vi "MegaAwesome_9_26_12a_JW.vi"() -> ()   [LabVIEW 2011]
uses:
  data/MegaAwesome_States.ctl
  <vilib>/Utility/inputDevices.llb/keyboardAcquire.vi
  <vilib>/Utility/file.llb/Read From Spreadsheet File (string).vi
  <vilib>/Utility/file.llb/Write To Spreadsheet File (string).vi
panel:
  out "Image Center X":i32
  in  "Disable Flag":bool
  out "Index":string
  out "ROI Descriptor out":T1 {"Contours"."Type" items=["No Selection", "Point", "Line", "Rectangle", "Oval", "Polygon", "Freehand Region", "Annulus", "Unused2", "Unused3", "Broken Line", "Freehand Line", "Rotated Rectangle"]}
  out "ROI Descriptor":T1 {"Contours"."Type" items=["No Selection", "Point", "Line", "Rectangle", "Oval", "Polygon", "Freehand Region", "Annulus", "Unused2", "Unused3", "Broken Line", "Freehand Line", "Rotated Rectangle"]}
  in  "Slider Min":dbl=5.0
  in  "Slider Max":dbl=5.0
  out "Opj X Axis":string
  out "X Axis Display Type":string
  in  "Index-Sat":dbl=5.0
  in  "Index-Lin":dbl=5.0
  in  "IndexLog-Lin":dbl=5.0
  in  "IndexLog-Sat":dbl=5.0 caption="Num Pts"
  out "Lin Id-Log Used":dbl[](array[numeric])
  out "Lin-Vg Array-Log Used":dbl[](array[numeric])
  in  "New: Comments":string
  out "Save Array":string[][](array[string])
  out "Folder Index":i32 caption="Length"
  out "Sat Id-Used":dbl[](array[numeric])
  out "Sat Vg Array-Used":dbl[](array[numeric])
  out "Vg Array-Log-Used":dbl[](array[numeric])
  out "Sat Id-Log-Used":dbl[](array[numeric])
  out "Lin Id-Used":dbl[](array[numeric])
  out "Lin-Vg Array-Used":dbl[](array[numeric])
  out "Lin Vd":dbl
  out "Recorded Prop":T2
  out "Current State":T3
  in  "Main Tab Control":T4(tab)
  in  "OE Link":bool
  in  "Transfer File":path
  out "Transfer Folder":path
  in  "1) Transport":bool caption="2) Transport"
  in  "Image Analysis":bool caption="1) Image Analysis"
  in  "Transport\nFolder":path caption="Transport Folder"
  out "Transport\nFile":path=path "D:/UserData/Desktop/Jeremy/WFU/Research/Programs/VI mods/Image Not Found.png" caption="Transport File"
  in  "Image Folder":path
  out "Image File":path=path "D:/UserData/Desktop/Jeremy/WFU/Research/Programs/VI mods/Image Not Found.png"
  out "Fabrication Prop":T5
  out "Distances":dbl[](array[numeric])
  in  "Zoom":i16(slide)=-3 scale=-5.0..5.0
  in  "Magnification":u16(ring) items=["5x", "10x", "20x", "50x", "80x"]
  in  "Undo Button":bool
  in  "Remove Button":bool
  in  "Transfer Plots":T6(tab)=enum."Saturation"
  in  "Lin-Trans Slider":dbl(slide) step=1.0 scale=-2.0..2.0 scale format="%#_1p"
  out "Sqrt-Lin":cluster{dbl[], dbl[]}[](graph)
  in  "Sat-Trans Slider":dbl(slide) step=1.0 scale=-2.0..2.0 scale format="%#_1p"
  out "Sqrt-Sat":cluster{dbl[], dbl[]}[](graph)
  out "Raw- Lin":cluster{dbl[], dbl[]}[](graph)
  out "Raw- Sat":cluster{dbl[], dbl[]}[](graph)
  in  "Log Plots":enum32{"Linear", "Saturation", "Transport"}(tab)=enum."Saturation"
  in  "Lin-Log Slider":dbl(slide) step=1.0 scale=-2.0..2.0 scale format="%#_1p"
  out "Lin-Log":cluster{dbl[], dbl[]}[](graph)
  in  "Sat-Log Slider":dbl(slide) step=1.0 scale=-2.0..2.0 scale format="%#_1p"
  out "Sat-Log":cluster{dbl[], dbl[]}[](graph)
  out "Transport":cluster{dbl[], dbl[]}[](graph)
  out "Transport Name:":string
  in  "Manual Controls":T7
  in  "File Controls":T8
  out "Date Recorded":string="Date Recorded" caption="Measured"
  out "Data Name:":string
  out "Image Name":string
  out "Date Created":string caption="Fabricated"
  in  "Comments:":string
  out "Rec: Length":dbl caption="Length" format="%#_3g"
  out "Rec: Width":dbl caption="Width" format="%#_4g"
  out "Rec: Dielectric (d)":dbl caption="Dielectric (d)" format="%#_3g"
  in  "New: Dielectric":dbl
  in  "New: Length":dbl
  in  "New: Width":dbl
  out "Rec: Temp":dbl caption="Sample Temp" format="%.1f"
  in  "New: Temp":dbl format="%.1f"
  out "Image Out":T9(plugin-control)
  in  "Num Pts":dbl=5.0
  in  "Num Pts Log":dbl=5.0 caption="Num Pts"
  out "Recorded Values Cluster":T10
  out "Calculated Values Cluster":T10 caption="Recorded Values Cluster"
  out "Re-Calculated Values Cluster":T10 caption="Recorded Values Cluster"
  in  "Independant Variable:":string(combo)="Length (um):"
  out "Image Preview":T9(plugin-control)
  out "Total Width":dbl
  in  "Index Array":u16(ring) caption="Index" items=["1A", "1A", "1A", "1A", "1A", "1A", "1A", "1A", "1A", "1A", "1A", "1A", "1A", "1A", "1A", "1A", "1A", "1A", "1A", "1A", "1A", "1A", "1A", "1A", "1A", "1A", "1A", "1A", "1A", "1A", "1A", "1A", "1A", "1A", "1A", "1A", "1A"]
  in  "Room Temp":dbl=294.0 caption="Room Temp (K)"
  out "No Image\n File":path=path "\\\\acad1\\physics/Jurchescu-group/JW-PD/Mega Awesome/Image Not Found.png" caption="No Image File"
  out "Origin Project File":path=path "\\\\acad1\\physics/Jurchescu-group/JW-PD/Group Library/Origin Project Files/DeviceData_8_10_12a_JW.opj"
  out "No Transport\n File":path=path "\\\\acad1\\physics/Jurchescu-group/JW-PD/Mega Awesome/No Transport File.txt" caption="No Transport File"
  in  "Transport Style Controls":T11={"Transport Line Size"=1, "Transport Line Color"=16772608} {"Transport Line Size" items=["Extra Small", "Small", "Medium", "Large", "Extra Large"]}
  out "Application Directory":path
  # "1)  Select the Transfer File that you would like to analyze:"
  # "Transfer Location"
  # "2) What else would you like to view during your analysis?"
  # "Transport Location"
  # "Image Location"
  # "Recorded"
  # "Calculated"
  # "Re-Calculated"
  # "Manual"
  # "um"
  # "Slider\nDoesn't\nWork"
  # "V"
  # "V"
  # "Slider\nDoesn't\nWork"
  # "V"
  # "Default File Choices"
  # "Default Analysis Values"
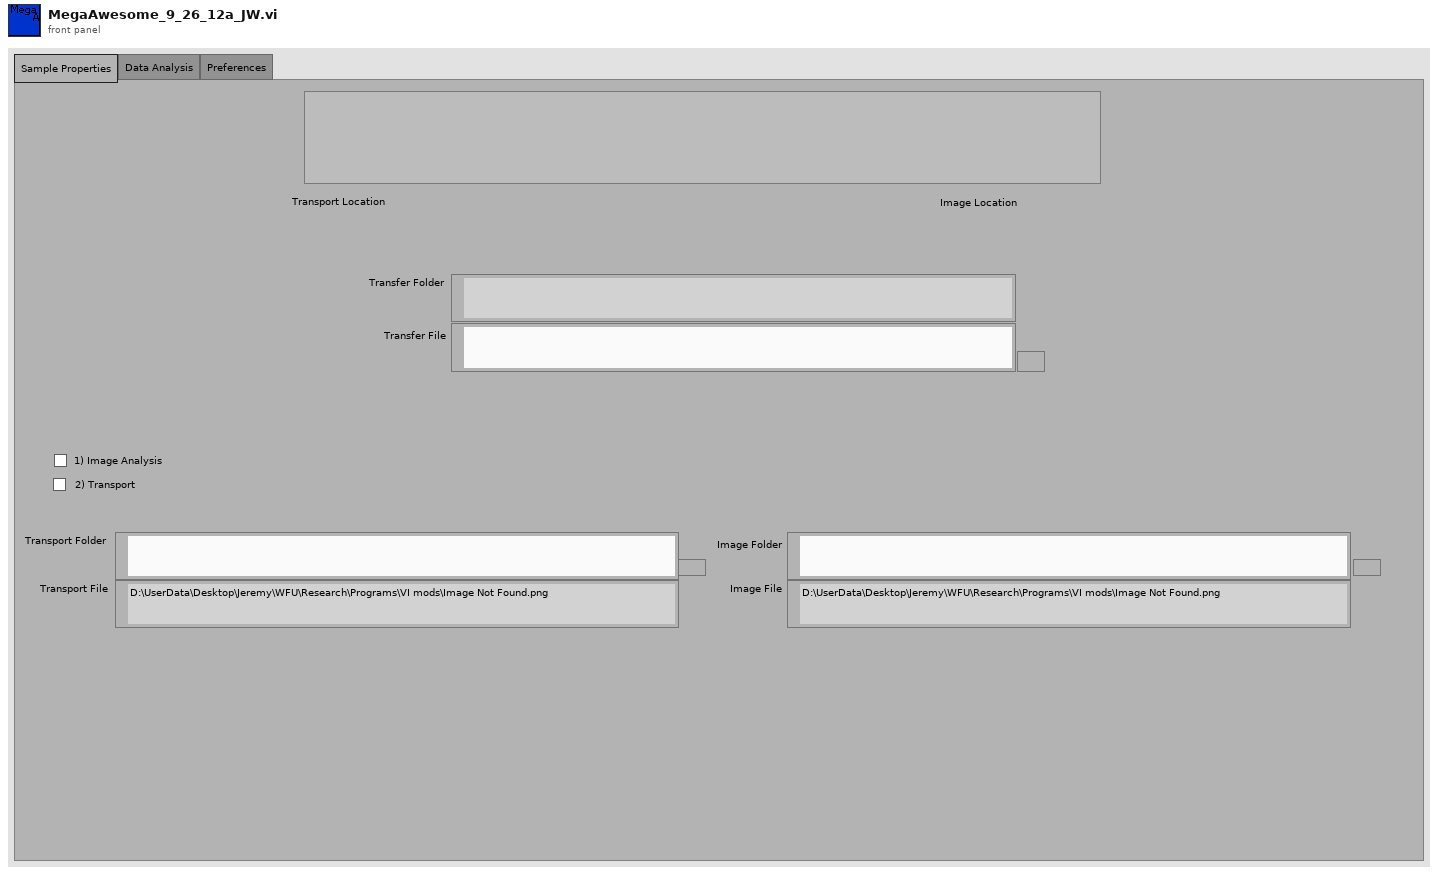
[diagram p1: front panel]
types:
  T1 = typedef "ROI Descriptor" = cluster{"Global Rectangle":i32[], "Contours":cluster{"ID":enum32{"External", "Internal"}, "Type":u32, "Coordinates":i32[]}[]}
  T2 = cluster{"Date Recorded":string, "Index":string, "Length":dbl, "Width":dbl, "Sample Temp":dbl}
  T3 = typedef "MegaAwesome_States.ctl" = enum16{"Init", "File Missing", "No Event", "Read Data", "Calculated Values", "Re-Calculated Values", "Next File", "Previous File", "Discard File", "Save", "Save Lines", "Export", "Exit"}
  T4 = enum32{"Sample Properties", "Data Analysis", "Preferences"}
  T5 = cluster{"Date Created":string, "Material":string, "Solvent":string, "Concentration":dbl, "Method":string, "Dielectric (nm)":dbl, "Treatment":string, "Comments":string}
  T6 = enum32{"Linear", "Saturation", "Raw-Linear", "Raw-Saturation"}
  T7 = cluster{"Manual-Temp":bool, "Manual-Width":bool, "Manuel-Length":bool, "Manuel-Dielectric":bool, "Manual Comments":bool}
  T8 = cluster{"Previous File":bool, "Discard ":bool, "Save Lines":bool, "Close":bool, "Next File ":bool, "Save":bool, "Save Next":bool, "Export":bool}
  T9 = typedef "IMAQ Image.ctl" = refnum<image>
  T10 = cluster{"Mobility-Sat":dbl, "Moblitity-Lin":dbl, "On/Off":dbl, "Off Current":dbl, "Vt-Sat":dbl, "STS":dbl, "Trap Density-VT":dbl, "Trap Density-STS":dbl}
  T11 = cluster{"Transport Line Size":u16, "Transport Line Color":u32}
  T12 = typedef "LVBoundsTypeDef.ctl" = cluster{"Width":u32, "Height":u32}
  T13 = cluster{"Global Rectangle":i32[], "Contours":cluster{"Contour Type":u32, "ROI Type":u32, "Points":i32[]}[]}
  T14 = cluster{"Contour Type":u32, "ROI Type":u32, "Points":i32[]}[]
  T15 = cluster{i32[], cluster{"Contour Type":u32, "ROI Type":u32, "Points":i32[]}[]}
  T16 = enum16{"0", "1", "2", "3", "4", "5", "6", "7", "8", "9", "A", "B", "C", "D", "E", "F", "G", "H", "I", "J", "K", "L", "M", "N", "O", "P", "Q", "R", "S", "T", "U", "V", "W", "X", "Y", "Z", "F1", "F2", "F3", "F4", "F5", "F6", "F7", "F8", "F9", "F10", "F11", "F12", "F13", "F14", "F15", "ADD", "BACK", "BACKSLASH", "CAPITAL", "COMMA", "DECIMAL", "DELETE", "DIVIDE", "DOWN", "END", "EQUALS", "ESCAPE", "GRAVE (`)", "HOME", "INSERT", "LBRACKET", "LCONTROL", "LEFT", "L ALT", "LSHIFT", "LWIN", "MINUS", "MULTIPLY", "NEXT", "NUMLOCK", "NUMPAD_0", "NUMPAD_1", "NUMPAD_2", "NUMPAD_3", "NUMPAD_4", "NUMPAD_5", "NUMPAD_6", "NUMPAD_7", "NUMPAD_8", "NUMPAD_9", "PAUSE", "PERIOD", "PRIOR (PG UP)", "RBRACKET", "RCONTROL", "RETURN", "RIGHT", "R ALT", "RSHIFT", "RWIN", "SCROLL", "SEMICOLON", "SLASH", "SPACE", "SUBTRACT", "TAB", "UP", "ENTER (num pad)", "' (quote)"}[]
  T17 = enum16{"0", "1", "2", "3", "4", "5", "6", "7", "8", "9", "A", "B", "C", "D", "E", "F", "G", "H", "I", "J", "K", "L", "M", "N", "O", "P", "Q", "R", "S", "T", "U", "V", "W", "X", "Y", "Z", "F1", "F2", "F3", "F4", "F5", "F6", "F7", "F8", "F9", "F10", "F11", "F12", "F13", "F14", "F15", "ADD", "BACK", "BACKSLASH", "CAPITAL", "COMMA", "DECIMAL", "DELETE", "DIVIDE", "DOWN", "END", "EQUALS", "ESCAPE", "GRAVE (`)", "HOME", "INSERT", "LBRACKET", "LCONTROL", "LEFT", "L ALT", "LSHIFT", "LWIN", "MINUS", "MULTIPLY", "NEXT", "NUMLOCK", "NUMPAD_0", "NUMPAD_1", "NUMPAD_2", "NUMPAD_3", "NUMPAD_4", "NUMPAD_5", "NUMPAD_6", "NUMPAD_7", "NUMPAD_8", "NUMPAD_9", "PAUSE", "PERIOD", "PRIOR (PG UP)", "RBRACKET", "RCONTROL", "RETURN", "RIGHT", "R ALT", "RSHIFT", "RWIN", "SCROLL", "SEMICOLON", "SLASH", "SPACE", "SUBTRACT", "TAB", "UP", "ENTER (num pad)", "' (quote)"}
  T18 = cluster{string, sgl, bool, bool, bool, bool, bool, bool, i32}
  T19 = cluster{i32, cluster{string, sgl, bool, bool, bool, bool, bool, bool, i32}, i32, i32}
  T20 = cluster{"Contour Type":u32, "ROI Type":u32, "Points":i32[]}
  T21 = cluster{"Points[0]":i32, "Points[1]":i32, "Points[2]":i32, "Points[3]":i32, "Points[4]":i32, "Points[5]":i32, "Points[6]":i32, "Points[7]":i32, "Points[8]":i32}
  T22 = cluster{"[0]":cluster{dbl[], dbl[]}, "[1]":cluster{dbl[], dbl[]}, "[2]":cluster{dbl[], dbl[]}, "[3]":cluster{dbl[], dbl[]}, "[4]":cluster{dbl[], dbl[]}, "[5]":cluster{dbl[], dbl[]}, "[6]":cluster{dbl[], dbl[]}, "[7]":cluster{dbl[], dbl[]}, "[8]":cluster{dbl[], dbl[]}}
  T23 = cluster{"Sat Vg Used":dbl[], "Sat Sqrt(Id) Used ":dbl[], "Lin Vg Used":dbl[], "Lin Sqrt(Id) Used":dbl[], "Index-Lin":dbl, "Index-Sat":dbl}
  T24 = cluster{"Raw Sat":cluster{dbl[], dbl[]}[], "Sqrt Sat":cluster{dbl[], dbl[]}[], "Log Sat":cluster{dbl[], dbl[]}[], "Raw Lin":cluster{dbl[], dbl[]}[], "Sqrt Lin":cluster{dbl[], dbl[]}[], "Log Lin":cluster{dbl[], dbl[]}[]}
  T25 = cluster{"Mobility-Sat":dbl, "Vt-Sat":dbl, "Mobility-Lin":dbl, "Vt-Lin":dbl, "Off I-Sat":dbl, "On/Off I-Sat":dbl}
  T26 = cluster{"Sat Vg Used":dbl[], "Sat Log(Id) Used":dbl[], "Lin Vg Used":dbl[], "Lin Log(Id) Used":dbl[], "STS Index-Sat":dbl, "STS Index-Lin":dbl}
  T27 = cluster{"Independant  Variable Indicator":string, "Parameter String Indicator":string}
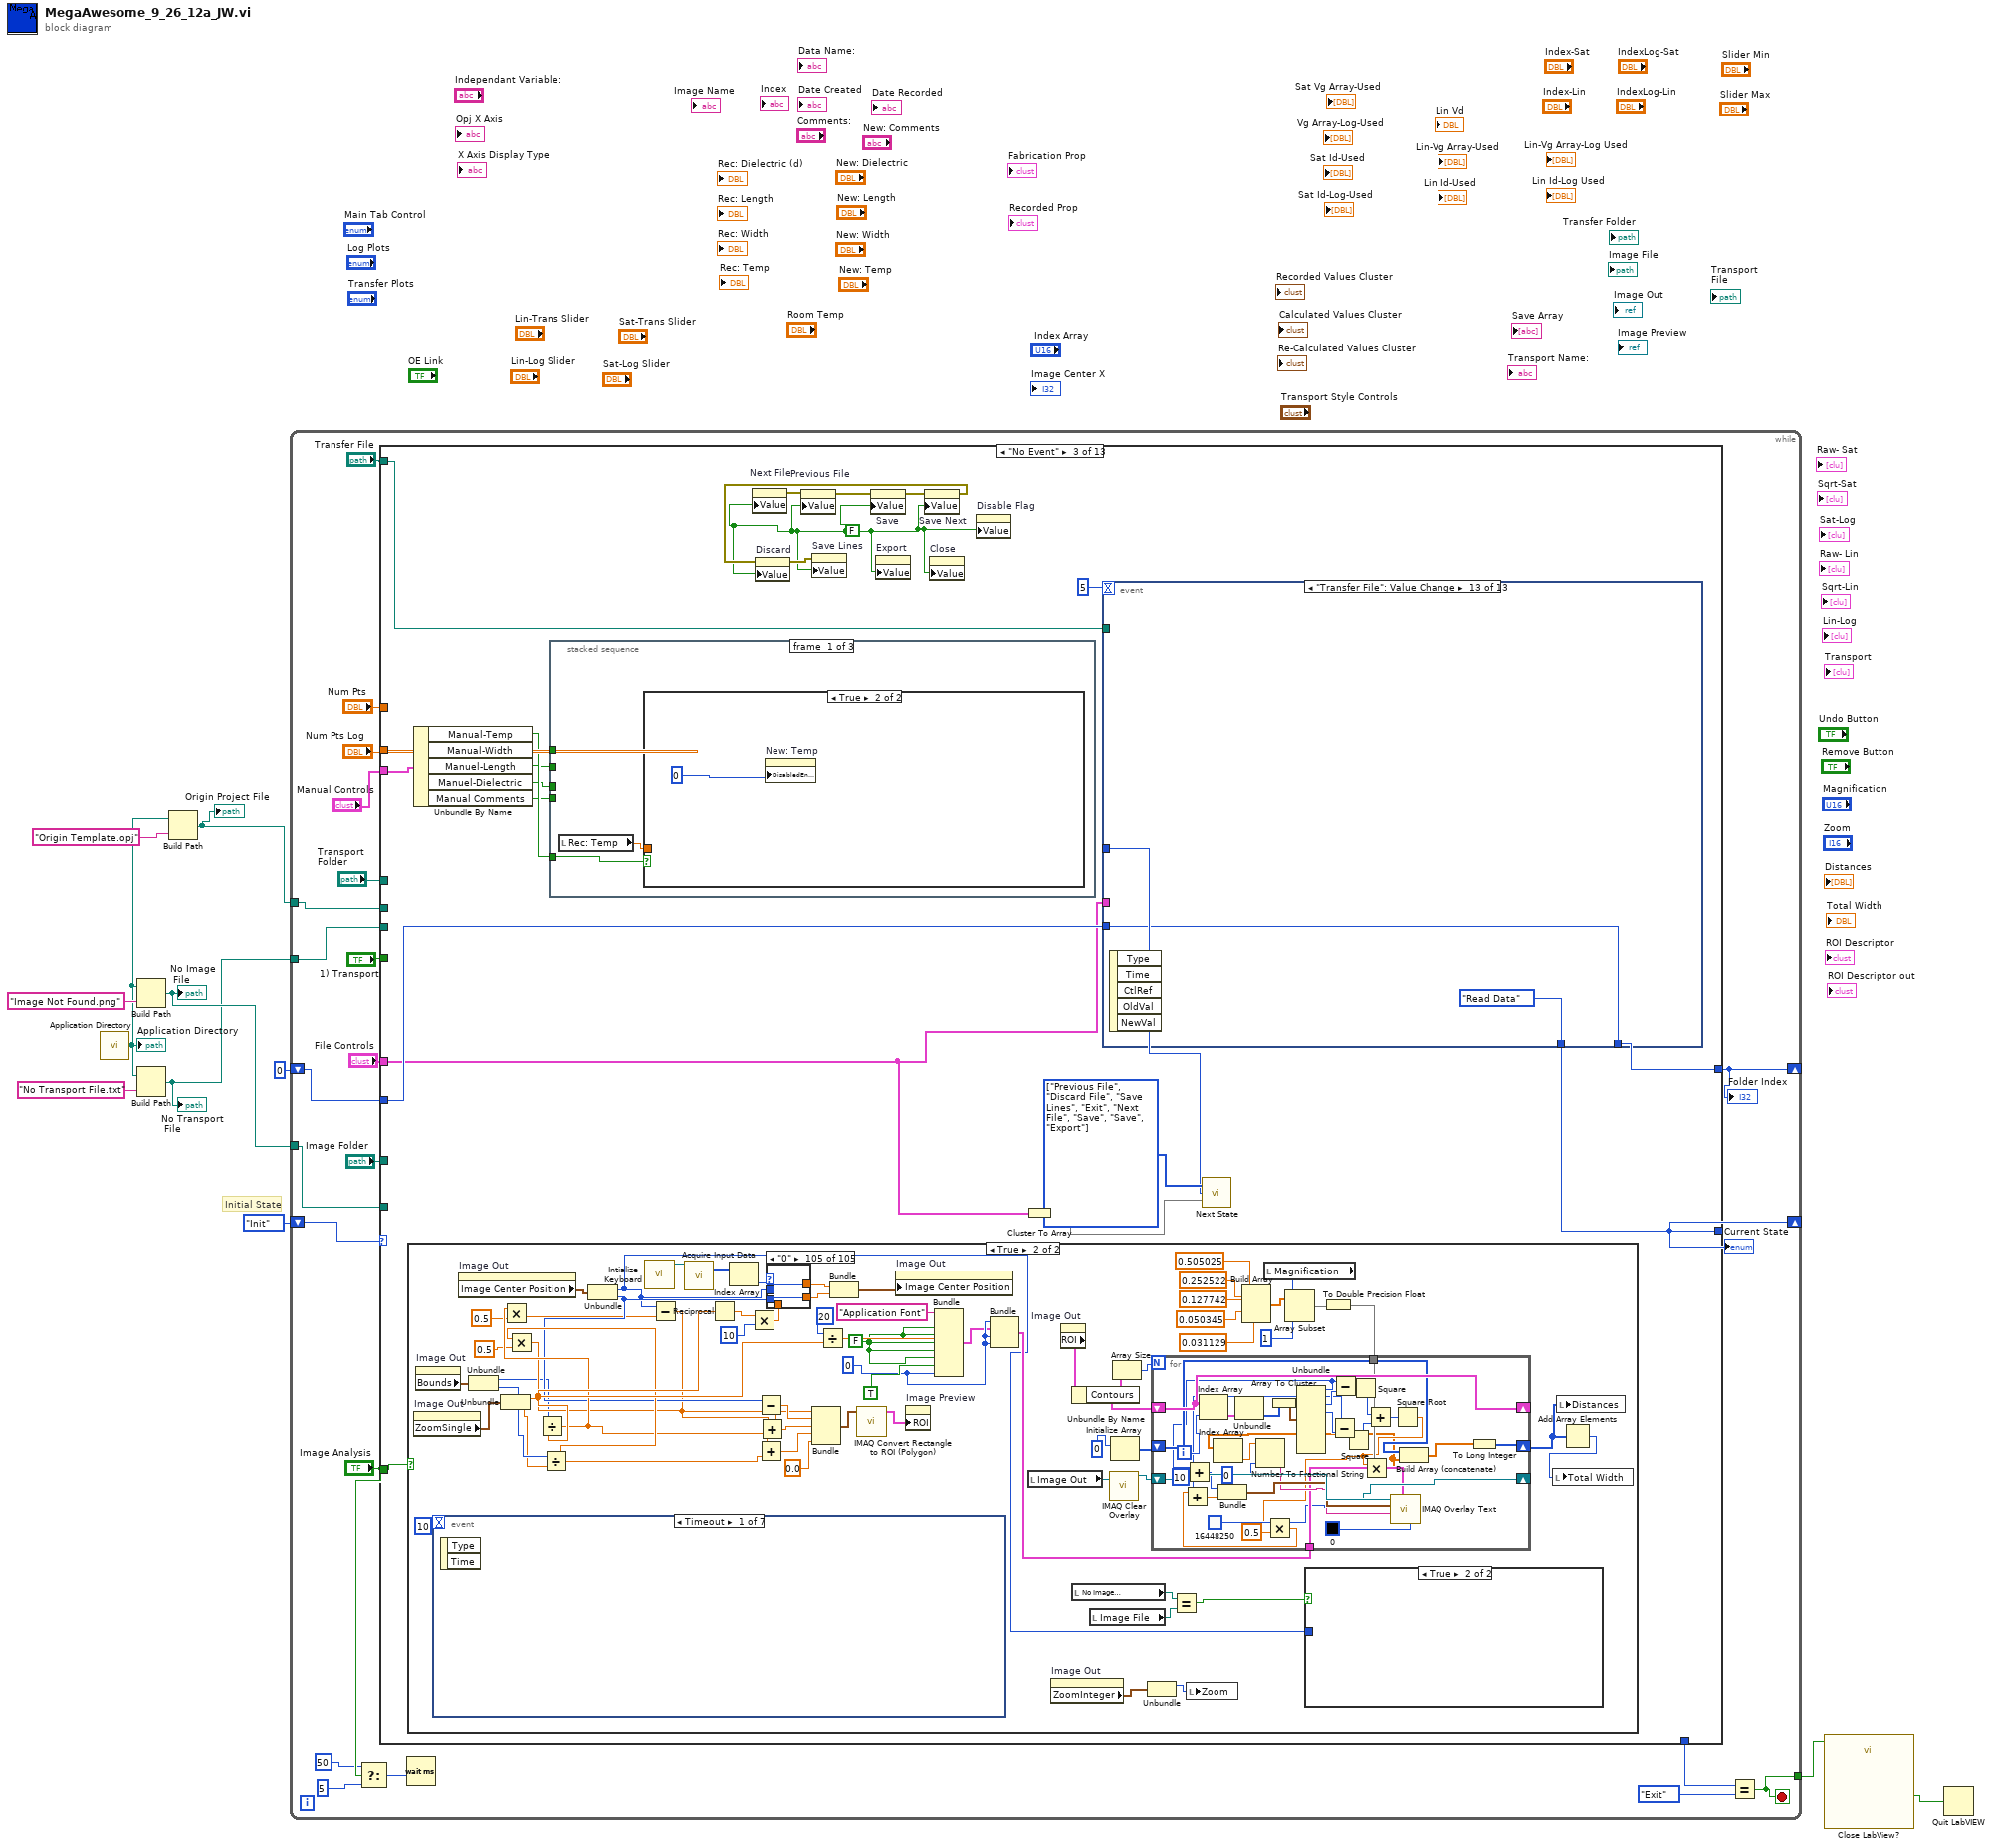
[diagram p0: block diagram]
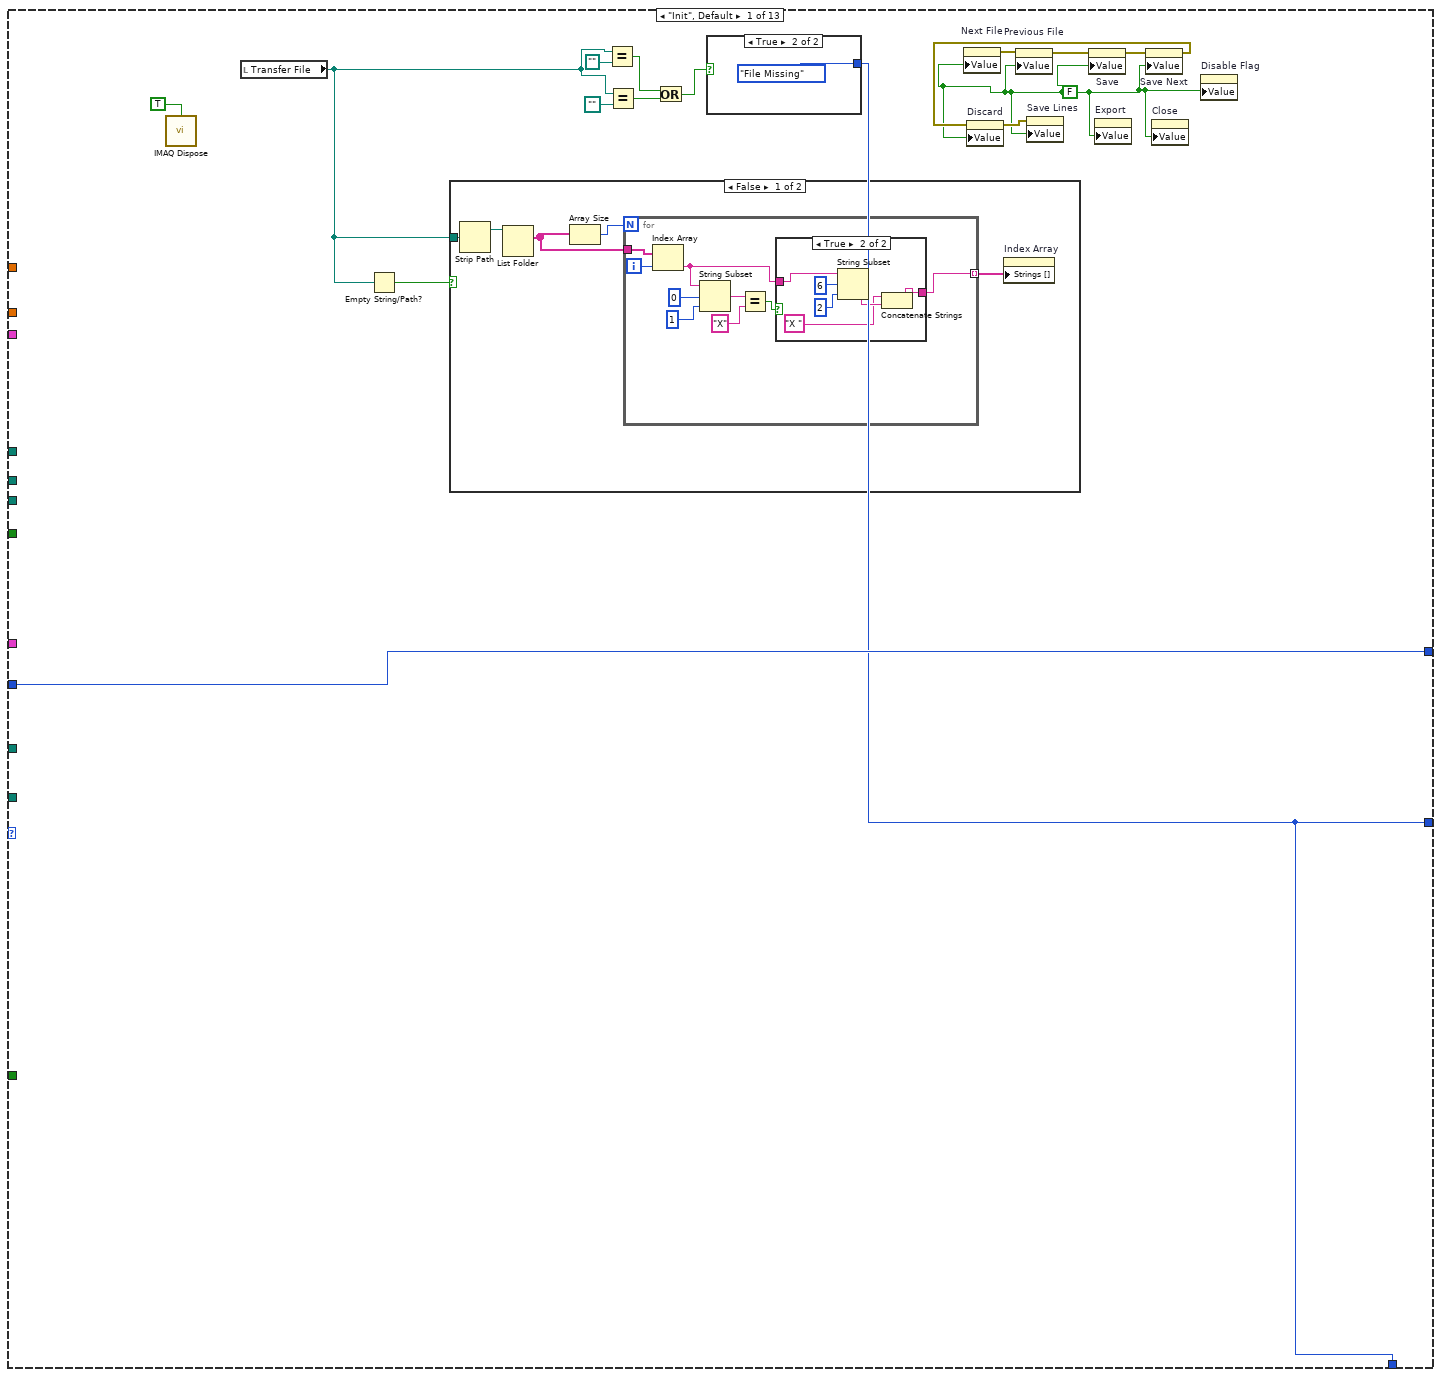
[diagram p2: hidden frame]
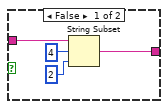
[diagram p3: hidden frame]
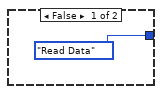
[diagram p5: hidden frame]
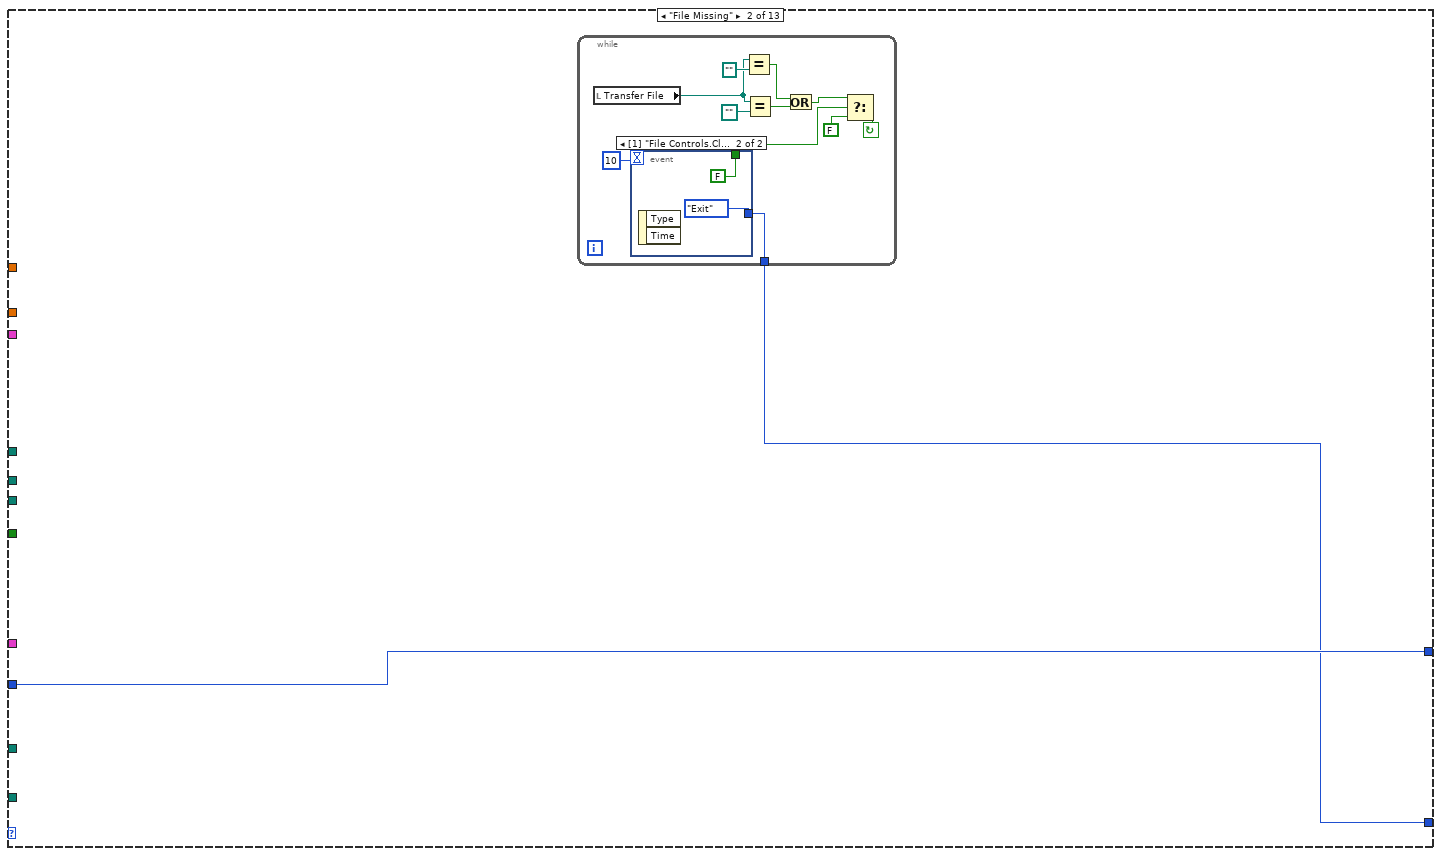
[diagram p6: hidden frame]
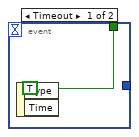
[diagram p7: hidden frame]
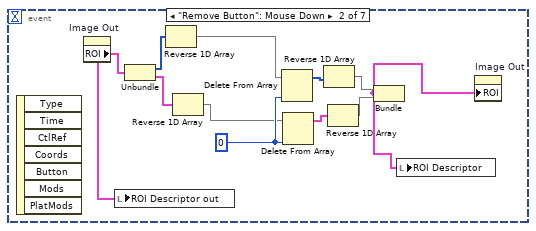
[diagram p9: hidden frame]
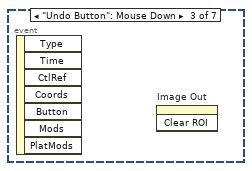
[diagram p10: hidden frame]
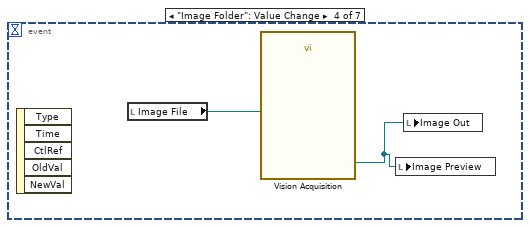
[diagram p11: hidden frame]
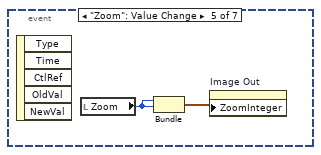
[diagram p12: hidden frame]
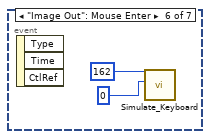
[diagram p13: hidden frame]
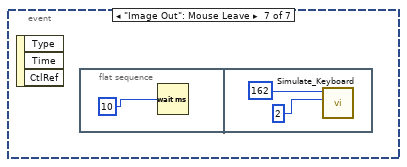
[diagram p14: hidden frame]
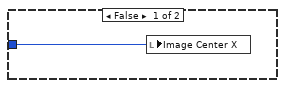
[diagram p15: hidden frame]
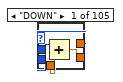
[diagram p16: hidden frame]
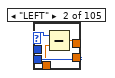
[diagram p17: hidden frame]
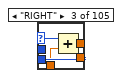
[diagram p18: hidden frame]
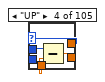
[diagram p19: hidden frame]
diagram:
  # "Initial State"
  n1 = call <vilib>:"Application Directory.vi"() -> ("Application Directory"=w4:path)
  "Application Directory" <- w4
  n2 = Build Path(base path=w4, name or relative path="Image Not Found.png") -> (appended path=w7:path)
  "No Image\n File" <- w7
  n3 = Build Path(base path=w4, name or relative path="No Transport File.txt") -> (appended path=w6:path)
  "No Transport\n File" <- w6
  n4 = Build Path(base path=w4, name or relative path="Origin Template.opj") -> (appended path=w5:path)
  "Origin Project File" <- w5
  n5 = while {
    shift-right: [w15] -> _
    shift-left: MegaAwesome_States."Init" -> [w13]
    shift-right: [w27] -> _
    shift-left: 0 -> [w28]
    tunnel: w7 -> [w19]
    tunnel: w6 -> [w17]
    tunnel: w5 -> [w16]
    tunnel: [w14] -> w2
    stop <- w14 stop-if-true
    n6 = Select(t=50, s="Image Analysis", f=5) -> (s? t:f=w21:i32)
    n7 = case shown="\"No Event\"" w13 {
      tunnel: [w34 w76 w104 MegaAwesome_States."Calculated Values" MegaAwesome_States."Re-Calculated Values" MegaAwesome_States."No Event" MegaAwesome_States."Read Data" MegaAwesome_States."Read Data" MegaAwesome_States."Init" w839 w1360 MegaAwesome_States."No Event" MegaAwesome_States."Exit"] -> w15
      tunnel: "Transfer File" -> [_ _ w94 w612 w659 _ w780 w791 w809 w844 _ _ _]
      tunnel: "Num Pts" -> [_ _ _ _ w683 _ _ _ _ _ _ _ _]
      tunnel: "Num Pts Log" -> [_ _ _ _ w682 _ _ _ _ _ _ _ _]
      tunnel: "Image Folder" -> [_ _ _ _ w679 _ _ _ _ _ _ w1371 _]
      tunnel: w19 -> [_ _ _ _ w678 _ _ _ _ _ _ _ _]
      tunnel: [w44 w77 w95 w617 w677 w740 w766 w789 w804 w845 w1361 w1381 w1386] -> w27
      tunnel: w28 -> [w44 w77 w96 w615 w677 w740 w767 w790 _ w845 w1361 w1381 w1386]
      tunnel: "Manual Controls" -> [_ _ w106 _ _ _ _ _ _ w843 _ _ _]
      tunnel: "File Controls" -> [_ _ w92 _ _ _ _ _ _ w838 _ _ _]
      tunnel: "1) Transport" -> [_ _ _ _ w650 _ _ _ _ _ _ _ _]
      tunnel: "Image Analysis" -> [_ _ w97 _ w649 _ _ _ _ _ _ _ _]
      tunnel: "Transport\nFolder" -> [_ _ _ _ w648 _ _ _ _ _ _ _ _]
      tunnel: w17 -> [_ _ _ _ w647 _ _ _ _ _ _ _ _]
      tunnel: w16 -> [_ _ _ _ _ _ _ _ _ _ _ _ w1385]
      tunnel: [w34 _ _ _ _ _ _ _ _ _ w1359 _ _] -> w12
      frame "Init", Default {
        w35 = FALSE
        n8 = call "IMAQ Dispose"("All Images? (No)"=TRUE) -> ()  [unwired: 5 in, 1 out]
        n9 = local read "Transfer File"() -> (w42:path)
        n10 = Empty String/Path?(string/path=w42) -> (empty?=w43:bool)
        n11 = case shown="False" w43 {
          tunnel: w42 -> [w51 _]
          frame False {
            n12 = Strip Path(path=w51) -> (stripped path=w53:path)  [unwired: 1 out]
            n13 = List Folder(path=w53) -> (filenames=w52:string[])  [unwired: 3 in, 3 out]
            n14 = Array Size(array=w52) -> (size(s)=w54:i32)
            n15 = for {
              N: w54 -> [_]
              tunnel: w52 -> [w63]
              tunnel: [w61] -> w50 mode=indexing
              i -> [w62]
              n16 = Index Array(array=w63, index=w62) -> (element=w60:string)
              n17 = String Subset(string=w60, offset (0)=0, length (rest)=1) -> (substring=w57:string)
              n18 = Equal?(x=w57, y="X") -> (x = y?=w56:bool)
              n19 = case shown="True" w56 {
                tunnel: w60 -> [w67 w71]
                tunnel: [w64 w70] -> w61
                frame False {
                  n20 = String Subset(string=w67, offset (0)=4, length (rest)=2) -> (substring=w64:string)
                }
                frame True {
                  n21 = String Subset(string=w71, offset (0)=6, length (rest)=2) -> (substring=w69:string)
                  n22 = Concatenate Strings("X ", w69) -> (w70:string)
                }
              }
            }
            n23 = property on="Index Array" class="Ring (strict)"("Strings []"=w50) -> ()  [unwired: 2 in, 2 out]
          }
          frame True {
          }
        }
        n24 = Equal?(x=w42, y=path "") -> (x = y?=w47:bool)
        n25 = Equal?(x=w42, y=path "") -> (x = y?=w46:bool)
        n26 = Or(x=w47, y=w46) -> (x .or. y?=w49:bool)
        n27 = case shown="True" w49 {
          tunnel: [MegaAwesome_States."Read Data" MegaAwesome_States."File Missing"] -> w34
          frame False {
          }
          frame True {
          }
        }
        n28 = property on="Next File" class="Bool (strict)"("Value"=w35) -> (error out=w40:errorcluster)  [unwired: 2 in, 1 out]
        n29 = property on="Previous File" class="Bool (strict)"(error in=w40, "Value"=w35) -> (error out=w39:errorcluster)  [unwired: 1 in, 1 out]
        n30 = property on="Save" class="Bool (strict)"(error in=w39, "Value"=w35) -> (error out=w38:errorcluster)  [unwired: 1 in, 1 out]
        n31 = property on="Export" class="Bool (strict)"("Value"=w35) -> ()  [unwired: 2 in, 2 out]
        n32 = property on="Save Next" class="Bool (strict)"(error in=w38, "Value"=w35) -> (error out=w37:errorcluster)  [unwired: 1 in, 1 out]
        n33 = property on="Discard" class="Bool (strict)"(error in=w37, "Value"=w35) -> (error out=w36:errorcluster)  [unwired: 1 in, 1 out]
        n34 = property on="Save Lines" class="Bool (strict)"(error in=w36, "Value"=w35) -> ()  [unwired: 1 in, 2 out]
        n35 = property on="Close" class="Bool (strict)"("Value"=w35) -> ()  [unwired: 2 in, 2 out]
        n36 = property on="Disable Flag" class="Bool (strict)"("Value"=w35) -> ()  [unwired: 2 in, 2 out]
      }
      frame "File Missing" {
        n37 = while {
          tunnel: [w83] -> w76
          stop <- w79 continue-if-true
          n38 = local read "Transfer File"() -> (w84:path)
          n39 = event shown="[1] \"File Controls.Close\": Value Change" {
            selector: _ -> [_ _]
            dyn-events: _ -> [_ _]
            timeout: 10 -> [_ _]
            tunnel: [_ MegaAwesome_States."Exit"] -> w83
            tunnel: [TRUE FALSE] -> w82
            event Timeout {
              n40 = event-data() -> ()  [unwired: 1 in, 2 out]
            }
            event "File Controls.Close": Value Change {
              n41 = event-data() -> ()  [unwired: 1 in, 2 out]
            }
          }
          n42 = Equal?(x=w84, y=path "") -> (x = y?=w86:bool)
          n43 = Equal?(x=w84, y=path "") -> (x = y?=w87:bool)
          n44 = Or(x=w86, y=w87) -> (x .or. y?=w81:bool)
          n45 = Select(t=w81, s=w82, f=FALSE) -> (s? t:f=w79:bool)
        }
      }
      frame "No Event" {
        w93 = FALSE
        w113 = T3[] [enum."Previous File", enum."Discard File", enum."Save Lines", enum."Exit", enum."Next File", enum."Save", enum."Save", enum."Export"] items=["Init", "File Missing", "No Event", "Read Data", "Calculated Values", "Re-Calculated Values", "Next File", "Previous File", "Discard File", "Save", "Save Lines", "Export", "Exit"]
        n46 = case shown="True" w97 {
          frame False {
          }
          frame True {
            w169 = FALSE
            w171 = 0
            n47 = property on="Image Out" class="ImageControl"() -> ("ZoomSingle"=w155:cluster{"X":sgl, "Y":sgl})  [unwired: 2 in, 2 out]
            n48 = property on="Image Out" class="ImageControl"() -> ("Bounds"=w154:T12)  [unwired: 2 in, 2 out]
            n49 = event shown="[0] Timeout" {
              selector: _ -> [_ _ _ _ _ _ _]
              dyn-events: _ -> [_ _ _ _ _ _ _]
              timeout: 10 -> [_ _ _ _ _ _ _]
              event Timeout {
                n50 = event-data() -> ()  [unwired: 1 in, 2 out]
              }
              event "Remove Button": Mouse Down {
                w188 = 0
                n51 = event-data() -> ()  [unwired: 1 in, 7 out]
                n52 = property on="Image Out" class="ImageControl"() -> ("ROI"=w178:T13)  [unwired: 2 in, 2 out]
                n53 = local write "ROI Descriptor out"(w178) -> ()
                n54 = Unbundle(w178) -> ("Global Rectangle"=w187:i32[], "Contours"=w185:T14)
                n55 = Reverse 1D Array(array=w187) -> (reversed array=w186:i32[])
                n56 = Reverse 1D Array(array=w185) -> (reversed array=w184:T14)
                n57 = Delete From Array(array=w186, index=w188) -> (array with subset deleted=w183:i32[])  [unwired: 1 in, 1 out]
                n58 = Delete From Array(array=w184, index=w188) -> (array with subset deleted=w182:T14)  [unwired: 1 in, 1 out]
                n59 = Reverse 1D Array(array=w183) -> (reversed array=w181:i32[])
                n60 = Reverse 1D Array(array=w182) -> (reversed array=w180:T14)
                n61 = Bundle(w181, w180) -> (w179:T15)  [unwired: 1 in]
                n62 = local write "ROI Descriptor"(w179) -> ()
                n63 = property on="Image Out" class="ImageControl"("ROI"=w179) -> ()  [unwired: 2 in, 2 out]
              }
              event "Undo Button": Mouse Down {
                n64 = event-data() -> ()  [unwired: 1 in, 7 out]
                n65 = invoke on="Image Out" class="ImageControl" method="Clear ROI"() -> ()  [unwired: 3 in, 3 out]
              }
              event "Image Folder": Value Change {
                n66 = event-data() -> ()  [unwired: 1 in, 5 out]
                n67 = local read "Image File"() -> (w190:path)
                n68 = call "Vision Acquisition"("Image Path"=w190) -> ("Image Out"=w189:T9)  [unwired: 25 in, 1 out]
                n69 = local write "Image Preview"(w189) -> ()
                n70 = local write "Image Out"(w189) -> ()
              }
              event "Zoom": Value Change {
                n71 = event-data() -> ()  [unwired: 1 in, 5 out]
                n72 = local read "Zoom"() -> (w191:i16)
                n73 = Bundle("Zoom"=w191, "Zoom"=w191) -> (w192:cluster{"Zoom":i16, "Zoom":i16})  [unwired: 1 in]
                n74 = property on="Image Out" class="ImageControl"("ZoomInteger"=w192) -> ()  [unwired: 2 in, 2 out]
              }
              event "Image Out": Mouse Enter {
                n75 = event-data() -> ()  [unwired: 1 in, 3 out]
                n76 = call "Simulate_Keyboard.vi"("Action"=0, "Virtual Key"=162) -> ()  [unwired: 7 in, 1 out]
              }
              event "Image Out": Mouse Leave {
                n77 = event-data() -> ()  [unwired: 1 in, 3 out]
                n78 = flat-sequence {
                  frame #0 {
                    n79 = Wait (ms)(milliseconds to wait=10) -> ()  [unwired: 1 out]
                  }
                  frame #1 {
                    n80 = call "Simulate_Keyboard.vi"("Action"=2, "Virtual Key"=162) -> ()  [unwired: 7 in, 1 out]
                  }
                }
              }
            }
            n81 = property on="Image Out" class="ImageControl"() -> ("Image Center Position"=w148:cluster{"X":u32, "Y":u32})  [unwired: 2 in, 2 out]
            n82 = Unbundle(w154) -> ("Width"=w157:u32, "Height"=w158:u32)
            n83 = Unbundle(w155) -> ("X"=w175:sgl, "Y"=w156:sgl)
            n84 = Divide(x=w157, y=w175) -> (x/y=w166:sgl)
            n85 = Multiply(x=w166, y=0.5) -> (x*y=w161:dbl)
            n86 = Divide(x=w158, y=w156) -> (x/y=w167:sgl)
            n87 = Multiply(x=w167, y=0.5) -> (x*y=w162:dbl)
            n88 = Unbundle(w148) -> ("X"=w118:u32, "Y"=w165:u32)
            n89 = call <vilib>:"Intialize Keyboard.vi"() -> ("device ID"=w145:refnum<k1>)  [unwired: 10 in, 1 out]
            n90 = Subtract(x=w118, y=w161) -> (x-y=w163:dbl)
            n91 = call-poly <vilib>:"Acquire Input Data.vi"("device ID"=w145) -> ("keys pressed"=w146:T16)  [unwired: 16 in, 2 out]
            n92 = Reciprocal(x=w175) -> (1/x=w176:sgl)
            n93 = Index Array(array=w146) -> (element=w142:T17)  [unwired: 1 in]
            n94 = Multiply(x=w176, y=10) -> (x*y=w174:sgl)
            n95 = Subtract(x=w165, y=w162) -> (x-y=w164:dbl)
            n96 = Add(x=w164, y=w167) -> (x+y=w150:dbl)
            n97 = Add(x=w163, y=w166) -> (x+y=w149:dbl)
            n98 = case shown="\"0\"" w142 {
              tunnel: w118 -> [w234 w240 w244 w246 w250 w252 w254 w256 w258 w260 w262 w264 w266 w268 w270 w272 w274 w276 w278 w280 w282 w284 w286 w288 w290 w292 w294 w296 w298 w300 w302 w304 w306 w308 w310 w312 w314 w316 w318 w320 w322 w324 w326 w328 w330 w332 w334 w336 w338 w340 w342 w344 w346 w348 w350 w352 w354 w356 w358 w360 w362 w364 w366 w368 w370 w372 w374 w376 w378 w380 w382 w384 w386 w388 w390 w392 w394 w396 w398 w400 w402 w404 w406 w408 w410 w412 w414 w416 w418 w420 w422 w424 w426 w428 w430 w432 w434 w436 w438 w440 w442 w444 w446 w448 w450]
              tunnel: [w234 w239 w243 w246 w250 w252 w254 w256 w258 w260 w262 w264 w266 w268 w270 w272 w274 w276 w278 w280 w282 w284 w286 w288 w290 w292 w294 w296 w298 w300 w302 w304 w306 w308 w310 w312 w314 w316 w318 w320 w322 w324 w326 w328 w330 w332 w334 w336 w338 w340 w342 w344 w346 w348 w350 w352 w354 w356 w358 w360 w362 w364 w366 w368 w370 w372 w374 w376 w378 w380 w382 w384 w386 w388 w390 w392 w394 w396 w398 w400 w402 w404 w406 w408 w410 w412 w414 w416 w418 w420 w422 w424 w426 w428 w430 w432 w434 w436 w438 w440 w442 w444 w446 w448 w450] -> w143
              tunnel: w165 -> [w236 w238 w242 w248 w249 w251 w253 w255 w257 w259 w261 w263 w265 w267 w269 w271 w273 w275 w277 w279 w281 w283 w285 w287 w289 w291 w293 w295 w297 w299 w301 w303 w305 w307 w309 w311 w313 w315 w317 w319 w321 w323 w325 w327 w329 w331 w333 w335 w337 w339 w341 w343 w345 w347 w349 w351 w353 w355 w357 w359 w361 w363 w365 w367 w369 w371 w373 w375 w377 w379 w381 w383 w385 w387 w389 w391 w393 w395 w397 w399 w401 w403 w405 w407 w409 w411 w413 w415 w417 w419 w421 w423 w425 w427 w429 w431 w433 w435 w437 w439 w441 w443 w445 w447 w449]
              tunnel: [w235 w238 w242 w247 w249 w251 w253 w255 w257 w259 w261 w263 w265 w267 w269 w271 w273 w275 w277 w279 w281 w283 w285 w287 w289 w291 w293 w295 w297 w299 w301 w303 w305 w307 w309 w311 w313 w315 w317 w319 w321 w323 w325 w327 w329 w331 w333 w335 w337 w339 w341 w343 w345 w347 w349 w351 w353 w355 w357 w359 w361 w363 w365 w367 w369 w371 w373 w375 w377 w379 w381 w383 w385 w387 w389 w391 w393 w395 w397 w399 w401 w403 w405 w407 w409 w411 w413 w415 w417 w419 w421 w423 w425 w427 w429 w431 w433 w435 w437 w439 w441 w443 w445 w447 w449] -> w144
              tunnel: w174 -> [w233 w237 w241 w245 _ _ _ _ _ _ _ _ _ _ _ _ _ _ _ _ _ _ _ _ _ _ _ _ _ _ _ _ _ _ _ _ _ _ _ _ _ _ _ _ _ _ _ _ _ _ _ _ _ _ _ _ _ _ _ _ _ _ _ _ _ _ _ _ _ _ _ _ _ _ _ _ _ _ _ _ _ _ _ _ _ _ _ _ _ _ _ _ _ _ _ _ _ _ _ _ _ _ _ _ _]
              frame "DOWN" {
                n99 = Add(x=w236, y=w233) -> (x+y=w235:sgl)
              }
              frame "LEFT" {
                n100 = Subtract(x=w240, y=w237) -> (x-y=w239:sgl)
              }
              frame "RIGHT" {
                n101 = Add(x=w244, y=w241) -> (x+y=w243:sgl)
              }
              frame "UP" {
                n102 = Subtract(x=w248, y=w245) -> (x-y=w247:sgl)
              }
              frame "ENTER (num pad)" {
              }
              frame "' (quote)" {
              }
              frame "END" {
              }
              frame "EQUALS" {
              }
              frame "ESCAPE" {
              }
              frame "GRAVE (`)" {
              }
              frame "HOME" {
              }
              frame "INSERT" {
              }
              frame "LBRACKET" {
              }
              frame "LCONTROL" {
              }
              frame "L ALT" {
              }
              frame "LSHIFT" {
              }
              frame "LWIN" {
              }
              frame "MINUS" {
              }
              frame "MULTIPLY" {
              }
              frame "NEXT" {
              }
              frame "NUMLOCK" {
              }
              frame "NUMPAD_0" {
              }
              frame "NUMPAD_1" {
              }
              frame "NUMPAD_2" {
              }
              frame "NUMPAD_3" {
              }
              frame "NUMPAD_4" {
              }
              frame "NUMPAD_5" {
              }
              frame "NUMPAD_6" {
              }
              frame "NUMPAD_7" {
              }
              frame "NUMPAD_8" {
              }
              frame "NUMPAD_9" {
              }
              frame "PAUSE" {
              }
              frame "PERIOD" {
              }
              frame "PRIOR (PG UP)" {
              }
              frame "RBRACKET" {
              }
              frame "RCONTROL" {
              }
              frame "RETURN" {
              }
              frame "R ALT" {
              }
              frame "RSHIFT" {
              }
              frame "RWIN" {
              }
              frame "SCROLL" {
              }
              frame "SEMICOLON" {
              }
              frame "SLASH" {
              }
              frame "SPACE" {
              }
              frame "SUBTRACT" {
              }
              frame "TAB" {
              }
              frame "DIVIDE" {
              }
              frame "DELETE" {
              }
              frame "DECIMAL" {
              }
              frame "COMMA" {
              }
              frame "CAPITAL" {
              }
              frame "BACKSLASH" {
              }
              frame "BACK" {
              }
              frame "ADD" {
              }
              frame "F15" {
              }
              frame "F14" {
              }
              frame "F13" {
              }
              frame "F12" {
              }
              frame "F11" {
              }
              frame "F10" {
              }
              frame "F9" {
              }
              frame "F8" {
              }
              frame "F7" {
              }
              frame "F6" {
              }
              frame "F5" {
              }
              frame "F4" {
              }
              frame "F3" {
              }
              frame "F2" {
              }
              frame "F1" {
              }
              frame "Z" {
              }
              frame "Y" {
              }
              frame "X" {
              }
              frame "W" {
              }
              frame "V" {
              }
              frame "U" {
              }
              frame "T" {
              }
              frame "S" {
              }
              frame "R" {
              }
              frame "Q" {
              }
              frame "P" {
              }
              frame "O" {
              }
              frame "N" {
              }
              frame "M" {
              }
              frame "L" {
              }
              frame "K" {
              }
              frame "J" {
              }
              frame "I" {
              }
              frame "H" {
              }
              frame "G" {
              }
              frame "F" {
              }
              frame "E" {
              }
              frame "D" {
              }
              frame "C" {
              }
              frame "B" {
              }
              frame "A" {
              }
              frame "9" {
              }
              frame "8" {
              }
              frame "7" {
              }
              frame "6" {
              }
              frame "5" {
              }
              frame "4" {
              }
              frame "3" {
              }
              frame "2" {
              }
              frame "1" {
              }
              frame "0" {
              }
            }
            n103 = Bundle(w163, w164, w149, w150, 0.0) -> (w151:cluster{dbl, dbl, dbl, dbl, dbl})  [unwired: 1 in]
            n104 = Divide(x=20, y=w175) -> (x/y=w173:sgl)
            n105 = Bundle("X"=w143, "Y"=w144) -> (w147:cluster{"X":sgl, "Y":sgl})  [unwired: 1 in]
            n106 = call "IMAQ Convert Rectangle to ROI (Polygon)"("Rectangle"=w151) -> ("ROI Descriptor"=w153:T1)  [unwired: 7 in, 2 out]
            n107 = property on="Image Out" class="ImageControl"("Image Center Position"=w147) -> ()  [unwired: 2 in, 2 out]
            n108 = property on="Image Preview" class="ImageControl"("ROI"=w153) -> ()  [unwired: 2 in, 2 out]
            n109 = Bundle("Application Font", w173, w169, w169, w169, w169, w169, TRUE, w171) -> (w168:T18)  [unwired: 1 in]
            n110 = Bundle(w171, w168, w171, w171) -> (w123:T19)  [unwired: 1 in]
            n111 = local read "Image Out"() -> (w122:T9)
            n112 = property on="Image Out" class="ImageControl"() -> ("ZoomInteger"=w121:cluster{"X":i32, "Y":i32})  [unwired: 2 in, 2 out]
            n113 = property on="Image Out" class="ImageControl"() -> ("ROI"=w126:T13)  [unwired: 2 in, 2 out]
            n114 = Unbundle By Name(w126) -> ("Contours"=w127:T14)
            n115 = local read "No Image\n File"() -> (w117:path)
            n116 = local read "Image File"() -> (w116:path)
            n117 = call "IMAQ Clear Overlay"("Image"=w122) -> ("Image Out"=w141:T9)  [unwired: 9 in, 1 out]
            n118 = Initialize Array(0) -> (w129:i32[])  [unwired: 1 in]
            n119 = Array Size(array=w127) -> (size(s)=w128:i32)
            n120 = Unbundle(w121) -> ("X"=w120:i32)  [unwired: 1 out]
            n121 = Equal?(x=w117, y=w116) -> (x = y?=w115:bool)
            n122 = local write "Zoom"(w120) -> ()
            n123 = Build Array(0.505025, 0.252522, 0.127742, 0.050345, 0.031129) -> (w136:dbl[])
            n124 = local read "Magnification"() -> (w137:u16)
            n125 = Array Subset(array=w136, index=w137, length=1) -> (w139:dbl[])
            n126 = case shown="True" w115 {
              tunnel: w118 -> [w198 _]
              frame False {
                n127 = local write "Image Center X"(w198) -> ()
              }
              frame True {
              }
            }
            n128 = To Double Precision Float(number=w139) -> (double precision float=w140:dbl[])
            n129 = for {
              N: w128 -> [_]
              shift-right: [w223] -> _
              shift-left: w127 -> [w223]
              shift-right: [w199] -> w124
              shift-left: w129 -> [w221]
              tunnel: w140 -> [w220]
              shift-right: [w217] -> _
              shift-left: w141 -> [w219]
              tunnel: w123 -> [w213]
              i -> [w216]
              n130 = Index Array(array=w223, index=w216) -> (element=w232:T20)
              n131 = Unbundle(w232) -> ("Points"=w231:i32[])  [unwired: 2 out]
              n132 = Array To Cluster(array=w231) -> (cluster=w230:T21)
              n133 = Unbundle(w230) -> ("Points[0]"=w212:i32, "Points[1]"=w209:i32, "Points[2]"=w222:i32, "Points[3]"=w228:i32)  [unwired: 5 out]
              n134 = Add(x=w212, y=10) -> (x+y=w210:i32)
              n135 = Subtract(x=w209, y=w228) -> (x-y=w227:i32)
              n136 = Subtract(x=w212, y=w222) -> (x-y=w229:i32)
              n137 = Square(x=w227) -> (x^2=w225:i32)
              n138 = Square(x=w229) -> (x^2=w226:i32)
              n139 = Add(x=w226, y=w225) -> (x+y=w224:i32)
              n140 = Square Root(x=w224) -> (sqrt(x)=w203:dbl)
              n141 = Multiply(x=w203, y=0.5) -> (x*y=w206:dbl)
              n142 = Add(x=w206, y=w209) -> (x+y=w208:dbl)
              n143 = Bundle(w210, w208) -> (w218:cluster{i32, dbl})  [unwired: 1 in]
              n144 = Multiply(x=w203, y=w220) -> (x*y=w202:dbl[])
              n145 = Index Array(array=w202) -> (element=w215:dbl)  [unwired: 1 in]
              n146 = Number To Fractional String(number=w215, precision (6)=0) -> (F-format string=w214:string)  [unwired: 2 in]
              n147 = call "IMAQ Overlay Text"("BG Color (Transparent)"=u32 0, "Text Color (black)"=u32 16448250, "Font, Size & Style"=w213, "String"=w214, "Origin"=w218, "Image"=w219) -> ("Image Out"=w217:T9)  [unwired: 4 in, 1 out]
              n148 = Build Array (concatenate)(w221, w202) -> (w200:dbl[])
              n149 = To Long Integer(number=w200) -> (32bit integer=w199:i32[])
            }
            n150 = local write "Distances"(w124) -> ()
            n151 = Add Array Elements(numeric array=w124) -> (sum=w125:i32)
            n152 = local write "Total Width"(w125) -> ()
          }
        }
        n153 = Unbundle By Name(w106) -> ("Manual-Temp"=w111:bool, "Manual-Width"=w110:bool, "Manuel-Length"=w109:bool, "Manuel-Dielectric"=w108:bool, "Manual Comments"=w107:bool)
        n154 = stacked-sequence {
          tunnel: w111 -> [w573 _ _]
          tunnel: w110 -> [_ w582 _]
          tunnel: w109 -> [_ _ w598]
          tunnel: w108 -> [_ _ w595]
          tunnel: w107 -> [_ _ w594]
          frame #0 {
            n155 = local read "Rec: Temp"() -> (w572:dbl)
            n156 = case shown="True" w573 {
              tunnel: w572 -> [w578 _]
              frame False {
                n157 = local read "Rec: Temp"() -> (w576:dbl)
                n158 = property on="New: Temp" class="DigNum (strict)"("DisabledEnum"=1) -> ()  [unwired: 2 in, 2 out]
                n159 = Equal To 0?(x=w576) -> (x = 0?=w577:bool)
                n160 = local write "New: Temp"(w578) -> ()
                n161 = case shown="True" w577 {
                  tunnel: [w579 w580] -> w574
                  tunnel: w576 -> [w579 _]
                  frame False {
                  }
                  frame True {
                    n162 = local read "Room Temp"() -> (w580:dbl)
                  }
                }
                n163 = local write "Rec: Temp"(w574) -> ()
                n164 = local write "New: Temp"(w574) -> ()
              }
              frame True {
                n165 = property on="New: Temp" class="DigNum (strict)"("DisabledEnum"=0) -> ()  [unwired: 2 in, 2 out]
              }
            }
          }
          frame #1 {
            n166 = case shown="True" w582 {
              frame False {
                n167 = property on="New: Width" class="DigNum (strict)"("DisabledEnum"=1) -> ()  [unwired: 2 in, 2 out]
              }
              frame True {
                n168 = property on="New: Width" class="DigNum (strict)"("DisabledEnum"=0) -> ()  [unwired: 2 in, 2 out]
              }
            }
            n169 = local read "Total Width"() -> (w588:dbl)
            n170 = Equal To 0?(x=w588) -> (x = 0?=w585:bool)
            n171 = local read "Rec: Width"() -> (w586:dbl)
            n172 = Not(x=w582) -> (.not. x?=w584:bool)
            n173 = Or(x=w585, y=w582) -> (x .or. y?=w587:bool)
            n174 = And(x=w585, y=w584) -> (x .and. y?=w583:bool)
            n175 = case shown="True" w583 {
              tunnel: w586 -> [_ w591]
              frame False {
              }
              frame True {
                n176 = local write "New: Width"(w591) -> ()
              }
            }
            n177 = case shown="True" w587 {
              tunnel: w588 -> [w592 _]
              frame False {
                n178 = local write "New: Width"(w592) -> ()
              }
              frame True {
                n179 = property on="New: Width" class="DigNum (strict)"("DisabledEnum"=0) -> ()  [unwired: 2 in, 2 out]
              }
            }
          }
          frame #2 {
            n180 = local read "Rec: Length"() -> (w599:dbl)
            n181 = case shown="False" w598 {
              tunnel: w599 -> [w607 _]
              frame False {
                n182 = local write "New: Length"(w607) -> ()
                n183 = property on="New: Length" class="DigNum (strict)"("DisabledEnum"=1) -> ()  [unwired: 2 in, 2 out]
              }
              frame True {
                n184 = property on="New: Length" class="DigNum (strict)"("DisabledEnum"=0) -> ()  [unwired: 2 in, 2 out]
              }
            }
            n185 = local read "Comments:"() -> (w596:string)
            n186 = local read "Rec: Dielectric (d)"() -> (w597:dbl)
            n187 = case shown="False" w594 {
              tunnel: w596 -> [w601 _]
              frame False {
                n188 = local write "New: Comments"(w601) -> ()
                n189 = property on="New: Comments" class="Str"("DisabledEnum"=1) -> ()  [unwired: 2 in, 2 out]
              }
              frame True {
                n190 = property on="New: Comments" class="Str"("DisabledEnum"=0) -> ()  [unwired: 2 in, 2 out]
              }
            }
            n191 = case shown="False" w595 {
              tunnel: w597 -> [w604 _]
              frame False {
                n192 = local write "New: Dielectric"(w604) -> ()
                n193 = property on="New: Dielectric" class="DigNum (strict)"("DisabledEnum"=1) -> ()  [unwired: 2 in, 2 out]
              }
              frame True {
                n194 = property on="New: Dielectric" class="DigNum (strict)"("DisabledEnum"=0) -> ()  [unwired: 2 in, 2 out]
              }
            }
          }
        }
        n195 = property on="Next File" class="Bool (strict)"("Value"=w93) -> (error out=w102:errorcluster)  [unwired: 2 in, 1 out]
        n196 = property on="Previous File" class="Bool (strict)"(error in=w102, "Value"=w93) -> (error out=w101:errorcluster)  [unwired: 1 in, 1 out]
        n197 = property on="Save" class="Bool (strict)"(error in=w101, "Value"=w93) -> (error out=w100:errorcluster)  [unwired: 1 in, 1 out]
        n198 = property on="Export" class="Bool (strict)"("Value"=w93) -> ()  [unwired: 2 in, 2 out]
        n199 = property on="Save Next" class="Bool (strict)"(error in=w100, "Value"=w93) -> (error out=w99:errorcluster)  [unwired: 1 in, 1 out]
        n200 = property on="Discard" class="Bool (strict)"(error in=w99, "Value"=w93) -> (error out=w98:errorcluster)  [unwired: 1 in, 1 out]
        n201 = property on="Save Lines" class="Bool (strict)"(error in=w98, "Value"=w93) -> ()  [unwired: 1 in, 2 out]
        n202 = property on="Close" class="Bool (strict)"("Value"=w93) -> ()  [unwired: 2 in, 2 out]
        n203 = property on="Disable Flag" class="Bool (strict)"("Value"=w93) -> ()  [unwired: 2 in, 2 out]
        n204 = Cluster To Array(cluster=w92) -> (array=w112:bool[])
        n205 = call "Next State.vi"("Buttons []"=w112, "States []"=w113) -> ("Enum"=w105:T3)
        n206 = event shown="[12] \"Transfer File\": Value Change" {
          selector: _ -> [_ _ _ _ _ _ _ _ _ _ _ _ _]
          dyn-events: _ -> [_ _ _ _ _ _ _ _ _ _ _ _ _]
          timeout: 5 -> [_ _ _ _ _ _ _ _ _ _ _ _ _]
          tunnel: w105 -> [w452 _ _ _ _ _ _ _ _ _ _ _ _]
          tunnel: [w452 MegaAwesome_States."Re-Calculated Values" MegaAwesome_States."Re-Calculated Values" MegaAwesome_States."Re-Calculated Values" MegaAwesome_States."Re-Calculated Values" MegaAwesome_States."Calculated Values" MegaAwesome_States."Re-Calculated Values" MegaAwesome_States."Re-Calculated Values" MegaAwesome_States."Calculated Values" MegaAwesome_States."Re-Calculated Values" MegaAwesome_States."Re-Calculated Values" MegaAwesome_States."Read Data" MegaAwesome_States."Read Data"] -> w104
          tunnel: w96 -> [w451 w453 w455 w457 w459 w461 w463 w488 w513 w518 w542 _ w570]
          tunnel: [w451 w453 w455 w457 w459 w461 w463 w488 w513 w518 w542 w561 w570] -> w95
          tunnel: w94 -> [_ _ _ _ _ _ _ _ _ _ _ w560 _]
          tunnel: w92 -> [_ _ _ _ _ _ _ _ _ _ _ _ _]
          event Timeout {
            n207 = event-data() -> ()  [unwired: 1 in, 2 out]
          }
          event "New: Dielectric": Value Change {
            n208 = event-data() -> ()  [unwired: 1 in, 5 out]
          }
          event "New: Length": Value Change {
            n209 = event-data() -> ()  [unwired: 1 in, 5 out]
          }
          event "New: Width": Value Change {
            n210 = event-data() -> ()  [unwired: 1 in, 5 out]
          }
          event "New: Temp": Value Change {
            n211 = event-data() -> ()  [unwired: 1 in, 5 out]
          }
          event "Num Pts Log", "Transport Style Controls", "Num Pts": Value Change {
            n212 = event-data() -> ()  [unwired: 1 in, 5 out]
          }
          event "Sat-Trans Slider": Value Change {
            n213 = event-data() -> ()  [unwired: 1 in, 5 out]
            n214 = local read "Sqrt-Sat"() -> (w487:cluster{dbl[], dbl[]}[])
            n215 = Decimate 1D Array(w487) -> (w471:cluster{dbl[], dbl[]}[], w472:cluster{dbl[], dbl[]}[])
            n216 = local read "Slider Min"() -> (w468:dbl)
            n217 = local read "Sat-Trans Slider"() -> (w466:dbl)
            n218 = Array To Cluster(array=w471) -> (cluster=w486:T22)
            n219 = local read "New: Dielectric"() -> (w481:dbl)
            n220 = local read "Num Pts"() -> (w464:dbl)
            n221 = local read "New: Width"() -> (w483:dbl)
            n222 = local read "New: Length"() -> (w482:dbl)
            n223 = Unbundle(w486) -> ("[0]"=w485:cluster{dbl[], dbl[]})  [unwired: 8 out]
            n224 = Absolute Value(x=w468) -> (abs(x)=w467:dbl)
            n225 = Unbundle(w485) -> (w469:dbl[], w484:dbl[])
            n226 = Add(x=w466, y=w467) -> (x+y=w465:dbl)
            n227 = Array Subset(array=w469, index=w465, length=w464) -> (w479:dbl[])
            n228 = local write "Sat Vg Array-Used"(w479) -> ()
            n229 = Array Subset(array=w484, index=w465, length=w464) -> (w480:dbl[])
            n230 = call "Mobility-Vt-Used Pts_Saturation.vi"("Width"=w483, "Length"=w482, "Dielectric (d)"=w481, "Sat Id Used"=w480, "Vg Used"=w479) -> ("Vt"=w475:dbl, "Mobility"=w476:dbl)  [unwired: 4 in, 1 out]
            n231 = local write "Index-Sat"(w465) -> ()
            n232 = local write "Sat Id-Used"(w480) -> ()
            n233 = Bundle(w479, w480) -> (w473:cluster{dbl[], dbl[]})  [unwired: 1 in]
            n234 = local read "Re-Calculated Values Cluster"() -> (w478:T10)
            n235 = Bundle By Name(cluster=w478, "Mobility-Sat"=w476, "Vt-Sat"=w475) -> (w477:T10)
            n236 = local write "Re-Calculated Values Cluster"(w477) -> ()
            n237 = Build Array (concatenate)(w471, w472, w473) -> (w470:cluster{dbl[], dbl[]}[])
            n238 = local write "Sqrt-Sat"(w470) -> ()
          }
          event "Lin-Trans Slider": Value Change {
            n239 = event-data() -> ()  [unwired: 1 in, 5 out]
            n240 = local read "Sqrt-Lin"() -> (w512:cluster{dbl[], dbl[]}[])
            n241 = Decimate 1D Array(w512) -> (w497:cluster{dbl[], dbl[]}[], w498:cluster{dbl[], dbl[]}[])
            n242 = local read "Slider Min"() -> (w494:dbl)
            n243 = Array To Cluster(array=w497) -> (cluster=w511:T22)
            n244 = local read "Lin-Trans Slider"() -> (w492:dbl)
            n245 = local read "New: Dielectric"() -> (w505:dbl)
            n246 = local read "Num Pts"() -> (w508:dbl)
            n247 = local read "New: Width"() -> (w507:dbl)
            n248 = local read "New: Length"() -> (w506:dbl)
            n249 = local read "Lin Vd"() -> (w489:dbl)
            n250 = Unbundle(w511) -> ("[0]"=w510:cluster{dbl[], dbl[]})  [unwired: 8 out]
            n251 = Absolute Value(x=w494) -> (abs(x)=w493:dbl)
            n252 = Unbundle(w510) -> (w495:dbl[], w509:dbl[])
            n253 = Add(x=w492, y=w493) -> (x+y=w491:dbl)
            n254 = Array Subset(array=w495, index=w491, length=w508) -> (w503:dbl[])
            n255 = local write "Lin-Vg Array-Used"(w503) -> ()
            n256 = Array Subset(array=w509, index=w491, length=w508) -> (w504:dbl[])
            n257 = call "Mobility-Vt-Used Pts_Linear.vi"("Width"=w507, "Length"=w506, "Vd"=w489, "Dielectric (d)"=w505, "Id Used"=w504, "Vg Used"=w503) -> ("Mobility"=w500:dbl)  [unwired: 3 in, 2 out]
            n258 = local write "Index-Lin"(w491) -> ()
            n259 = local write "Lin Id-Used"(w504) -> ()
            n260 = Bundle(w503, w504) -> (w499:cluster{dbl[], dbl[]})  [unwired: 1 in]
            n261 = local read "Re-Calculated Values Cluster"() -> (w502:T10)
            n262 = Bundle By Name(cluster=w502, "Moblitity-Lin"=w500) -> (w501:T10)
            n263 = local write "Re-Calculated Values Cluster"(w501) -> ()
            n264 = Build Array (concatenate)(w497, w498, w499) -> (w496:cluster{dbl[], dbl[]}[])
            n265 = local write "Sqrt-Lin"(w496) -> ()
          }
          event "Image Analysis", "1) Transport": Value Change {
            n266 = event-data() -> ()  [unwired: 1 in, 5 out]
          }
          event "Sat-Log Slider": Value Change {
            n267 = event-data() -> ()  [unwired: 1 in, 5 out]
            n268 = local read "Sat-Log"() -> (w521:cluster{dbl[], dbl[]}[])
            n269 = property on="Sat-Log" class="XYGraph (strict)"("Active Plot"=2, "Plot.Fill/Pt. Color"=u32 6618880, "Plot.Point Style"=11) -> ()  [unwired: 2 in, 2 out]
            n270 = Decimate 1D Array(w521) -> (w528:cluster{dbl[], dbl[]}[], w529:cluster{dbl[], dbl[]}[])
            n271 = local read "Slider Min"() -> (w525:dbl)
            n272 = Array To Cluster(array=w528) -> (cluster=w538:T22)
            n273 = local read "Num Pts Log"() -> (w535:dbl)
            n274 = local read "Sat-Log Slider"() -> (w523:dbl)
            n275 = Unbundle(w538) -> ("[0]"=w537:cluster{dbl[], dbl[]})  [unwired: 8 out]
            n276 = Absolute Value(x=w525) -> (abs(x)=w524:dbl)
            n277 = Unbundle(w537) -> (w526:dbl[], w536:dbl[])
            n278 = Add(x=w523, y=w524) -> (x+y=w520:dbl)
            n279 = Array Subset(array=w526, index=w520, length=w535) -> (w533:dbl[])
            n280 = Array Subset(array=w536, index=w520, length=w535) -> (w534:dbl[])
            n281 = local write "Vg Array-Log-Used"(w533) -> ()
            n282 = local write "IndexLog-Sat"(w520) -> ()
            n283 = Bundle(w533, w534) -> (w519:cluster{dbl[], dbl[]})  [unwired: 1 in]
            n284 = call "STS-Used.vi"("Id Used"=w534, "Vg-Used"=w533) -> ("STS"=w530:dbl)  [unwired: 9 in]
            n285 = local write "Sat Id-Log-Used"(w534) -> ()
            n286 = local read "Re-Calculated Values Cluster"() -> (w532:T10)
            n287 = Bundle By Name(cluster=w532, "STS"=w530) -> (w531:T10)
            n288 = local write "Re-Calculated Values Cluster"(w531) -> ()
            n289 = Build Array (concatenate)(w528, w529, w519) -> (w527:cluster{dbl[], dbl[]}[])
            n290 = local write "Sat-Log"(w527) -> ()
          }
          event "Lin-Log Slider": Value Change {
            # "No Indicator for Lin-Log Slider Use"
            n291 = event-data() -> ()  [unwired: 1 in, 5 out]
            n292 = local read "Lin-Log"() -> (w546:cluster{dbl[], dbl[]}[])
            n293 = property on="Lin-Log" class="XYGraph (strict)"("Active Plot"=2, "Plot.Fill/Pt. Color"=u32 6618880, "Plot.Point Style"=11) -> ()  [unwired: 2 in, 2 out]
            n294 = Decimate 1D Array(w546) -> (w552:cluster{dbl[], dbl[]}[], w553:cluster{dbl[], dbl[]}[])
            n295 = local read "Slider Min"() -> (w549:dbl)
            n296 = Array To Cluster(array=w552) -> (cluster=w559:T22)
            n297 = local read "Num Pts Log"() -> (w556:dbl)
            n298 = local read "Lin-Log Slider"() -> (w547:dbl)
            n299 = Unbundle(w559) -> ("[0]"=w558:cluster{dbl[], dbl[]})  [unwired: 8 out]
            n300 = Absolute Value(x=w549) -> (abs(x)=w548:dbl)
            n301 = Unbundle(w558) -> (w550:dbl[], w557:dbl[])
            n302 = Add(x=w547, y=w548) -> (x+y=w545:dbl)
            n303 = Array Subset(array=w550, index=w545, length=w556) -> (w554:dbl[])
            n304 = local write "Lin-Vg Array-Log Used"(w554) -> ()
            n305 = Array Subset(array=w557, index=w545, length=w556) -> (w555:dbl[])
            n306 = local write "IndexLog-Sat"(w545) -> ()
            n307 = Bundle(w554, w555) -> (w544:cluster{dbl[], dbl[]})  [unwired: 1 in]
            n308 = local write "Lin Id-Log Used"(w555) -> ()
            n309 = Build Array (concatenate)(w552, w553, w544) -> (w551:cluster{dbl[], dbl[]}[])
            n310 = local write "Lin-Log"(w551) -> ()
          }
          event "Index Array": Value Change {
            n311 = event-data() -> ()  [unwired: 1 in, 5 out]
            n312 = Strip Path(path=w560) -> (stripped path=w566:path)  [unwired: 1 out]
            n313 = local write "Transfer Folder"(w566) -> ()
            n314 = List Folder(path=w566) -> (filenames=w562:string[])  [unwired: 3 in, 3 out]
            n315 = local read "Index Array"() -> (w561:u16)
            n316 = Path To String(path=w566) -> (string=w567:string)
            n317 = Index Array(array=w562, index=w561) -> (element=w568:string)
            n318 = Concatenate Strings(w567, "\\", w568) -> (w564:string)
            n319 = String To Path(string=w564) -> (path=w563:path)
            n320 = local write "Transfer File"(w563) -> ()
          }
          event "Transfer File": Value Change {
            n321 = event-data() -> ()  [unwired: 1 in, 5 out]
          }
        }
      }
      frame "Read Data" {
        n322 = call "IMAQ Dispose"("All Images? (No)"=TRUE) -> ()  [unwired: 5 in, 1 out]
        n323 = case shown="False" "Disable Flag" {
          tunnel: w615 -> [_ w642]
          tunnel: [w638 w639] -> w614
          tunnel: w612 -> [w638 _]
          frame False {
          }
          frame True {
            n324 = local read "Transfer Folder"() -> (w641:path)
            n325 = List Folder(path=w641) -> (filenames=w643:string[])  [unwired: 3 in, 3 out]
            n326 = Index Array(array=w643, index=w642) -> (element=w640:string)
            n327 = Build Path(base path=w641, name or relative path=w640) -> (appended path=w639:path)
            n328 = local write "Transfer File"(w639) -> ()
          }
        }
        n329 = call "Recorded Values.vi"("Path"=w614) -> ("Recorded Char"=w637:T10, "Recorded Prop"=w628:T2, "Fabrication Prop"=w626:T5)  [unwired: 8 in]
        n330 = Strip Path(path=w614) -> (stripped path=w625:path, name=w624:string)
        n331 = local write "Fabrication Prop"(w626) -> ()
        n332 = local write "Recorded Prop"(w628) -> ()
        n333 = Unbundle By Name(w628) -> ("Date Recorded"=w610:string, "Index"=w627:string, "Length"=w620:dbl, "Width"=w619:dbl)  [unwired: 1 out]
        n334 = local write "Recorded Values Cluster"(w637) -> ()
        n335 = Unbundle By Name(w628) -> ("Sample Temp"=w630:dbl)
        n336 = Unbundle By Name(w626) -> ("Dielectric (nm)"=w621:dbl, "Comments"=w622:string, "Date Created"=w611:string)
        n337 = List Folder(path=w625) -> (filenames=w618:string[])  [unwired: 3 in, 3 out]
        n338 = local write "Rec: Dielectric (d)"(w621) -> ()
        n339 = local write "Date Created"(w611) -> ()
        n340 = local write "Index"(w627) -> ()
        n341 = local write "Rec: Length"(w620) -> ()
        n342 = local write "Rec: Width"(w619) -> ()
        n343 = Equal To 0?(x=w630) -> (x = 0?=w633:bool)
        n344 = Number To Decimal String(number=w630) -> (decimal integer string=w634:string)  [unwired: 1 in]
        n345 = local write "Comments:"(w622) -> ()
        n346 = Search 1D Array(1D array=w618, element=w624) -> (index of element=w617:i32)  [unwired: 1 in]
        n347 = Equal?(x="", y=w634) -> (x = y?=w632:bool)
        n348 = Index Array(array=w618, index=w617) -> (element=w623:string)
        n349 = local write "New: Width"(w619) -> ()
        n350 = local write "New: Length"(w620) -> ()
        n351 = local write "Index Array"(w617) -> ()
        n352 = local write "Date Recorded"(w610) -> ()
        n353 = Or(x=w633, y=w632) -> (x .or. y?=w631:bool)
        n354 = local write "New: Dielectric"(w621) -> ()
        n355 = local write "Data Name:"(w623) -> ()
        n356 = case shown="True" w631 {
          tunnel: [w644 w645] -> w609
          tunnel: w630 -> [w644 _]
          frame False {
          }
          frame True {
            n357 = local read "Room Temp"() -> (w645:dbl)
          }
        }
        n358 = local write "New: Temp"(w609) -> ()
        n359 = Bundle By Name(cluster=w628, "Sample Temp"=w609) -> (w629:T2)
        n360 = local write "Rec: Temp"(w609) -> ()
        n361 = local write "Recorded Prop"(w629) -> ()
      }
      frame "Calculated Values" {
        n362 = case shown="True" w650 {
          selector: w650 -> [w723 _]
          tunnel: w659 -> [w722 w734]
          tunnel: w648 -> [w721 w730]
          tunnel: w647 -> [w726 w728]
          frame False {
            n363 = call "TRF to TSP Plot_09_21_12a_JW.vi"("Plot Transport"=w723, "No Transport File"=w726, "Transport Folder"=w721, "Transfer File"=w722) -> ("Transport"=w724:cluster{ext[], ext[]}[], "Transport File"=w725:path, "Transport Name"=w720:string)  [unwired: 5 in]
            n364 = local write "Transport"(w724) -> ()
            n365 = local write "Transport\nFile"(w725) -> ()
            n366 = local write "Transport Name:"(w720) -> ()
          }
          frame True {
            n367 = local read "Transport Style Controls"() -> (w733:T11)
            n368 = call "TRF to TSP Plot_09_21_12a_JW.vi"("Transport Graph Properties"=w733, "No Transport File"=w728, "Transport Folder"=w730, "Transfer File"=w734) -> ("Transport"=w732:cluster{ext[], ext[]}[], "Transport File"=w729:path, "Transport Name"=w727:string)  [unwired: 5 in]
            n369 = Array Size(array=w732) -> (size(s)=w731:i32)
            n370 = local write "Transport"(w732) -> ()
            n371 = for {
              N: w731 -> [_]
              tunnel: w733 -> [w738]
              i -> [w737]
              n372 = Unbundle By Name(w738) -> ("Transport Line Size"=w735:u16, "Transport Line Color"=w736:u32)
              n373 = property on="Transport" class="XYGraph (strict)"("Active Plot"=w737, "Plot.Plot Color"=w736, "Plot.Line Width"=w735) -> ()  [unwired: 2 in, 2 out]
            }
            n374 = local write "Transport\nFile"(w729) -> ()
            n375 = local write "Transport Name:"(w727) -> ()
          }
        }
        n376 = case shown="True" w649 {
          tunnel: w679 -> [_ w708]
          tunnel: w678 -> [w700 w714]
          tunnel: w659 -> [_ w713]
          frame False {
            n377 = call "Vision Acquisition2"("Image Path"=w700) -> ("Image Out"=w699:T9)  [unwired: 25 in, 1 out]
            n378 = local write "Image Out"(w699) -> ()
            n379 = local write "Image Preview"(w699) -> ()
          }
          frame True {
            n380 = local read "Image Center X"() -> (w701:i32)
            n381 = call "Image from TRF Display.vi"("Image Center X"=w701, "No Image File"=w714, "Image Folder"=w708, "Transfer File"=w713) -> ("Image Preview"=w709:T9, "Image Out"=w710:T9, "Image File"=w711:path, "Image Name"=w712:string, "ROI File"=w705:path)  [unwired: 3 in]
            n382 = invoke on="Image Out" class="ImageControl" method="Clear ROI"() -> ()  [unwired: 3 in, 3 out]
            n383 = local write "Image File"(w711) -> ()
            n384 = local write "Image Name"(w712) -> ()
            n385 = local write "Image Out"(w710) -> ()
            n386 = local write "Image Preview"(w709) -> ()
            n387 = call <vilib>:"Check if File or Folder Exists.vi"("path"=w705) -> ("file or folder exists?"=w706:bool, "dup path"=w707:path)  [unwired: 8 in, 1 out]
            n388 = case shown="True" w706 {
              tunnel: w707 -> [_ w715]
              frame False {
              }
              frame True {
                n389 = Read from Text File(file (use dialog)=w715) -> (text=w719:string)  [unwired: 3 in, 3 out]
                n390 = property on="Image Out" class="ImageControl"() -> ("ROI"=w716:T13)  [unwired: 2 in, 2 out]
                n391 = Unflatten From String(type=w716, binary string=w719) -> (value=w717:T13, error out=w718:errorcluster)  [unwired: 3 in, 1 out]
                n392 = property on="Image Out" class="ImageControl"(error in=w718, "ROI"=w717) -> ()  [unwired: 1 in, 2 out]
              }
            }
            n393 = local read "Image Center X"() -> (w702:i32)
            n394 = Bundle("Image Center X"=w702, 0) -> (w704:cluster{"Image Center X":i32, i32})  [unwired: 1 in]
            n395 = property on="Image Out" class="ImageControl"("Image Center Position"=w704) -> ()  [unwired: 2 in, 2 out]
          }
        }
        n396 = local read "Recorded Prop"() -> (w681:T2)
        n397 = local read "Fabrication Prop"() -> (w688:T5)
        n398 = local read "Calculated Values Cluster"() -> (w698:T10)
        n399 = call "Mobility-Vt Calculator-File.vi"("NumPts"=w683, "Path"=w659) -> ("Used Points"=w676:T23, "Graph Cluster"=w665:T24, "Lin Vd"=w672:dbl, "Output"=w696:T25)  [unwired: 6 in]
        n400 = call "STS Calculator-File.vi"("NumPts"=w682, "Path"=w659) -> ("Used Points"=w670:T26, "XY Graph-Sat"=w653:cluster{dbl[], dbl[]}[], "XY Graph-Lin"=w646:cluster{dbl[], dbl[]}[], "Ouput"=w691:cluster{"STS-Sat":dbl, "STS-Lin":dbl})  [unwired: 6 in]
        n401 = Unbundle By Name(w688) -> ("Dielectric (nm)"=w686:dbl)
        n402 = Unbundle By Name(w681) -> ("Sample Temp"=w680:dbl)
        n403 = Unbundle By Name(w696) -> ("Mobility-Sat"=w695:dbl, "Vt-Sat"=w687:dbl, "Mobility-Lin"=w694:dbl, "Off I-Sat"=w693:dbl, "On/Off I-Sat"=w692:dbl)  [unwired: 1 out]
        n404 = local write "Lin Vd"(w672) -> ()
        n405 = Unbundle By Name(w691) -> ("STS-Sat"=w685:dbl)  [unwired: 1 out]
        n406 = local write "Sat-Log"(w653) -> ()
        n407 = local write "Lin-Log"(w646) -> ()
        n408 = call "Trap Density_VT.vi"("VT"=w687, "Dielectric"=w686) -> ("Trap Density-VT"=w690:dbl)
        n409 = call "Trap Density_STS.vi"("Temp (T) [K]"=w680, "S.T.S. (S)"=w685, "Dielectric"=w686) -> ("Trap Density (N)"=w689:dbl)  [unwired: 8 in]
        n410 = Bundle By Name(cluster=w698, "Mobility-Sat"=w695, "Moblitity-Lin"=w694, "On/Off"=w692, "Off Current"=w693, "Vt-Sat"=w687, "STS"=w685, "Trap Density-VT"=w690, "Trap Density-STS"=w689) -> (w697:T10)
        n411 = Unbundle By Name(w670) -> ("Sat Vg Used"=w669:dbl[], "Sat Log(Id) Used"=w668:dbl[], "Lin Vg Used"=w667:dbl[], "Lin Log(Id) Used"=w666:dbl[], "STS Index-Sat"=w651:dbl, "STS Index-Lin"=w652:dbl)
        n412 = Unbundle By Name(w676) -> ("Sat Vg Used"=w675:dbl[], "Sat Sqrt(Id) Used"=w674:dbl[], "Lin Vg Used"=w673:dbl[], "Lin Sqrt(Id) Used"=w671:dbl[], "Index-Lin"=w661:dbl, "Index-Sat"=w660:dbl)
        n413 = local write "Vg Array-Log-Used"(w669) -> ()
        n414 = local write "Sat Id-Log-Used"(w668) -> ()
        n415 = local write "Lin-Vg Array-Log Used"(w667) -> ()
        n416 = local write "Lin Id-Log Used"(w666) -> ()
        n417 = local write "IndexLog-Sat"(w651) -> ()
        n418 = local write "Index-Lin"(w652) -> ()
        n419 = local write "Calculated Values Cluster"(w697) -> ()
        n420 = local write "Sat Vg Array-Used"(w675) -> ()
        n421 = local write "Sat Id-Used"(w674) -> ()
        n422 = local write "Lin-Vg Array-Used"(w673) -> ()
        n423 = local write "Lin Id-Used"(w671) -> ()
        n424 = local write "Index-Sat"(w660) -> ()
        n425 = local write "Index-Lin"(w661) -> ()
        n426 = local write "Lin-Log Slider"(w652) -> ()
        n427 = local write "Sat-Log Slider"(w651) -> ()
        n428 = local write "Sat-Trans Slider"(w660) -> ()
        n429 = local write "Lin-Trans Slider"(w661) -> ()
        n430 = Unbundle By Name(w665) -> ("Raw Sat"=w658:cluster{dbl[], dbl[]}[], "Sqrt Sat"=w662:cluster{dbl[], dbl[]}[], "Raw Lin"=w664:cluster{dbl[], dbl[]}[], "Sqrt Lin"=w663:cluster{dbl[], dbl[]}[])
        n431 = Index Array(array=w658) -> (element=w657:cluster{dbl[], dbl[]})  [unwired: 1 in]
        n432 = Unbundle(w657) -> (w656:dbl[])  [unwired: 1 out]
        n433 = Array Max & Min(array=w656) -> (max value=w655:dbl, min value=w654:dbl)  [unwired: 2 out]
        n434 = property on="Sat-Trans Slider" class="Slide (strict)"("Scale.Maximum"=w655, "Scale.Minimum"=w654) -> ()  [unwired: 2 in, 2 out]
        n435 = property on="Lin-Trans Slider" class="Slide (strict)"("Scale.Maximum"=w655, "Scale.Minimum"=w654) -> ()  [unwired: 2 in, 2 out]
        n436 = property on="Sat-Log Slider" class="Slide (strict)"("Scale.Maximum"=w655, "Scale.Minimum"=w654) -> ()  [unwired: 2 in, 2 out]
        n437 = property on="Lin-Log Slider" class="Slide (strict)"("Scale.Maximum"=w655, "Scale.Minimum"=w654) -> ()  [unwired: 2 in, 2 out]
        n438 = local write "Slider Max"(w655) -> ()
        n439 = local write "Slider Min"(w654) -> ()
        n440 = local write "Raw- Sat"(w658) -> ()
        n441 = local write "Raw- Lin"(w664) -> ()
        n442 = local write "Sqrt-Sat"(w662) -> ()
        n443 = local write "Sqrt-Lin"(w663) -> ()
      }
      frame "Re-Calculated Values" {
        n444 = local read "Vg Array-Log-Used"() -> (w747:dbl[])
        n445 = local read "Sat Vg Array-Used"() -> (w755:dbl[])
        n446 = local read "Lin-Vg Array-Used"() -> (w761:dbl[])
        n447 = local read "Sat Id-Log-Used"() -> (w746:dbl[])
        n448 = local read "New: Dielectric"() -> (w759:dbl)
        n449 = local read "New: Dielectric"() -> (w744:dbl)
        n450 = local read "New: Length"() -> (w758:dbl)
        n451 = local read "New: Length"() -> (w754:dbl)
        n452 = local read "New: Width"() -> (w757:dbl)
        n453 = local read "New: Width"() -> (w753:dbl)
        n454 = local read "Lin Id-Used"() -> (w760:dbl[])
        n455 = local read "Sat Id-Used"() -> (w752:dbl[])
        n456 = local read "Re-Calculated Values Cluster"() -> (w763:T10)
        n457 = local read "New: Dielectric"() -> (w743:dbl)
        n458 = local read "New: Temp"() -> (w742:dbl)
        n459 = local read "Lin Vd"() -> (w739:dbl)
        n460 = call "Mobility-Vt-Used Pts_Saturation.vi"("Width"=w753, "Length"=w754, "Dielectric (d)"=w744, "Sat Id Used"=w752, "Vg Used"=w755) -> ("Vt"=w750:dbl, "Mobility"=w751:dbl)  [unwired: 4 in, 1 out]
        n461 = call "STS-Used.vi"("Id Used"=w746, "Vg-Used"=w747) -> ("STS"=w745:dbl)  [unwired: 9 in]
        n462 = call "Mobility-Vt-Used Pts_Linear.vi"("Width"=w757, "Length"=w758, "Vd"=w739, "Dielectric (d)"=w759, "Id Used"=w760, "Vg Used"=w761) -> ("Mobility"=w756:dbl)  [unwired: 3 in, 2 out]
        n463 = call "Trap Density_VT.vi"("VT"=w750, "Dielectric"=w744) -> ("Trap Density-VT"=w749:dbl)
        n464 = call "Trap Density_STS.vi"("Temp (T) [K]"=w742, "S.T.S. (S)"=w745, "Dielectric"=w743) -> ("Trap Density (N)"=w741:dbl)  [unwired: 8 in]
        n465 = Bundle By Name(cluster=w763, "Mobility-Sat"=w751, "Moblitity-Lin"=w756, "Vt-Sat"=w750, "STS"=w745, "Trap Density-VT"=w749, "Trap Density-STS"=w741) -> (w762:T10)
        n466 = local write "Re-Calculated Values Cluster"(w762) -> ()
      }
      frame "Next File" {
        n467 = call "IMAQ Dispose"("All Images? (No)"=TRUE) -> ()  [unwired: 5 in, 1 out]
        n468 = Strip Path(path=w780) -> (stripped path=w771:path, name=w778:string)
        n469 = local write "Transfer Folder"(w771) -> ()
        n470 = List Folder(path=w771) -> (filenames=w765:string[])  [unwired: 3 in, 3 out]
        n471 = Array Size(array=w765) -> (size(s)=w777:i32)
        n472 = Search 1D Array(1D array=w765, element=w778) -> (index of element=w775:i32)  [unwired: 1 in]
        n473 = Decrement(x=w777) -> (x-1=w776:i32)
        n474 = Equal?(x=w776, y=w775) -> (x = y?=w774:bool)
        n475 = case shown="True" w774 {
          tunnel: w767 -> [w782 _]
          tunnel: [w781 0] -> w766
          frame False {
            n476 = Increment(x=w782) -> (x+1=w781:i32)
          }
          frame True {
          }
        }
        n477 = Path To String(path=w771) -> (string=w772:string)
        n478 = Index Array(array=w765, index=w766) -> (element=w773:string)
        n479 = Concatenate Strings(w772, "\\", w773) -> (w769:string)
        n480 = String To Path(string=w769) -> (path=w768:path)
        n481 = local write "Transfer File"(w768) -> ()
      }
      frame "Previous File" {
        n482 = call "IMAQ Dispose"("All Images? (No)"=TRUE) -> ()  [unwired: 5 in, 1 out]
        n483 = Strip Path(path=w791) -> (stripped path=w788:path, name=w799:string)
        n484 = local write "Transfer Folder"(w788) -> ()
        n485 = List Folder(path=w788) -> (filenames=w792:string[])  [unwired: 3 in, 3 out]
        n486 = Array Size(array=w792) -> (size(s)=w786:i32)
        n487 = Search 1D Array(1D array=w792, element=w799) -> (index of element=w798:i32)  [unwired: 1 in]
        n488 = Decrement(x=w786) -> (x-1=w785:i32)
        n489 = Equal To 0?(x=w798) -> (x = 0?=w797:bool)
        n490 = case shown="True" w797 {
          tunnel: w790 -> [w802 _]
          tunnel: [w801 w803] -> w789
          tunnel: w785 -> [_ w803]
          frame False {
            n491 = Decrement(x=w802) -> (x-1=w801:i32)
          }
          frame True {
          }
        }
        n492 = Path To String(path=w788) -> (string=w787:string)
        n493 = Index Array(array=w792, index=w789) -> (element=w796:string)
        n494 = Concatenate Strings(w787, "\\", w796) -> (w794:string)
        n495 = String To Path(string=w794) -> (path=w793:path)
        n496 = local write "Transfer File"(w793) -> ()
      }
      frame "Discard File" {
        n497 = flat-sequence {
          tunnel: w809 -> [w812]
          tunnel: [w812] -> w808
          tunnel: [w811] -> w805
          tunnel: w808 -> [w824]
          tunnel: w805 -> [w817]
          tunnel: [w816] -> w804
          frame #0 {
            n498 = Strip Path(path=w812) -> (stripped path=w815:path, name=w814:string)
            n499 = List Folder(path=w815) -> (filenames=w813:string[])  [unwired: 3 in, 3 out]
            n500 = Search 1D Array(1D array=w813, element=w814) -> (index of element=w811:i32)  [unwired: 1 in]
          }
          frame #1 {
            n501 = Strip Path(path=w824) -> (stripped path=w825:path, name=w823:string)
            n502 = String Subset(string=w823, offset (0)=0, length (rest)=1) -> (substring=w820:string)
            n503 = Equal?(x=w820, y="X") -> (x = y?=w818:bool)
            n504 = case shown="True" w818 {
              tunnel: w825 -> [w832 _]
              tunnel: w824 -> [w828 _]
              tunnel: w823 -> [w827 _]
              tunnel: w817 -> [w826 w836]
              tunnel: [w826 w835] -> w816
              frame False {
                n505 = Path To String(path=w832) -> (string=w831:string)
                n506 = Concatenate Strings(w831, "\\", "X_", w827) -> (w830:string)
                n507 = String To Path(string=w830) -> (path=w829:path)
                n508 = Move(source path=w828, 10:w829) -> ()  [unwired: 3 in, 3 out]
              }
              frame True {
                n509 = Increment(x=w836) -> (x+1=w835:i32)
              }
            }
          }
        }
        n510 = property on="Disable Flag" class="Bool (strict)"("Value"=TRUE) -> ()  [unwired: 2 in, 2 out]
        n511 = call "IMAQ Dispose"("All Images? (No)"=TRUE) -> ()  [unwired: 5 in, 1 out]
      }
      frame "Save" {
        n512 = stacked-sequence {
          seq-local: [w852 _] -> [_ w1349]
          seq-local: [w851 _] -> [_ w1347]
          tunnel: w844 -> [w853 w1350]
          frame #0 {
            # "Saves each Re-calculated parameter in sequence"
            n513 = stacked-sequence {
              tunnel: [_ _ _ _ _ _ _ _ _ _ _ _ _ w1317] -> w851
              tunnel: w853 -> [w873 _ _ _ _ _ _ _ _ _ _ _ _ _]
              frame #0 {
                n514 = call-poly <vilib>:"Read From Spreadsheet File.vi"("file path (dialog if empty)"=w873) -> ("all rows"=w872:string[][])  [unwired: 6 in, 4 out]
                n515 = Array Size(array=w872) -> (size(s)=w877:i32[])
                n516 = Array Subset(array=w872, index (row)=0, index (col)=0, length (col)=3) -> (w881:string[][])  [unwired: 1 in]
                n517 = Index Array(array=w877, index=0) -> (element=w875:i32)
                n518 = Reshape Array(w881, w875) -> (w874:string[])
                n519 = Search 1D Array(1D array=w874, element="Dielectric (nm):") -> (index of element=w884:i32)  [unwired: 1 in]
                n520 = Equal?(x=w884, y=-1) -> (x = y?=w883:bool)
                n521 = case shown="False" w883 {
                  tunnel: w872 -> [w892 w896]
                  tunnel: w884 -> [w888 _]
                  tunnel: [w887 w896] -> w882
                  frame False {
                    n522 = local read "Rec: Dielectric (d)"() -> (w894:dbl)
                    n523 = Number To Fractional String(number=w894) -> (F-format string=w889:string)  [unwired: 3 in]
                    n524 = Divide(x=w888, y=3) -> (x/y=w891:dbl)
                    n525 = To Word Integer(number=w891) -> (16bit integer=w890:i16)
                    n526 = Replace Array Subset(array=w892, new element=w889, index (row)=w890, index (col)=1) -> (w887:string[][])
                  }
                  frame True {
                  }
                }
                n527 = local write "Save Array"(w882) -> ()
              }
              frame #1 {
                n528 = local read "Save Array"() -> (w898:string[][])
                n529 = Array Size(array=w898) -> (size(s)=w901:i32[])
                n530 = Array Subset(array=w898, index (row)=0, index (col)=0, length (col)=3) -> (w905:string[][])  [unwired: 1 in]
                n531 = Index Array(array=w901, index=0) -> (element=w899:i32)
                n532 = Reshape Array(w905, w899) -> (w897:string[])
                n533 = Search 1D Array(1D array=w897, element="Comments:") -> (index of element=w908:i32)  [unwired: 1 in]
                n534 = Equal?(x=w908, y=-1) -> (x = y?=w907:bool)
                n535 = case shown="False" w907 {
                  tunnel: w898 -> [w916 w919]
                  tunnel: w908 -> [w913 _]
                  tunnel: [w912 w919] -> w906
                  frame False {
                    n536 = local read "New: Comments"() -> (w911:string)
                    n537 = Divide(x=w913, y=3) -> (x/y=w915:dbl)
                    n538 = To Word Integer(number=w915) -> (16bit integer=w914:i16)
                    n539 = Replace Array Subset(array=w916, new element=w911, index (row)=w914, index (col)=1) -> (w912:string[][])
                  }
                  frame True {
                  }
                }
                n540 = local write "Save Array"(w906) -> ()
              }
              frame #2 {
                n541 = local read "Save Array"() -> (w921:string[][])
                n542 = Array Size(array=w921) -> (size(s)=w924:i32[])
                n543 = Array Subset(array=w921, index (row)=0, index (col)=0, length (col)=3) -> (w928:string[][])  [unwired: 1 in]
                n544 = Index Array(array=w924, index=0) -> (element=w922:i32)
                n545 = Reshape Array(w928, w922) -> (w920:string[])
                n546 = Search 1D Array(1D array=w920, element="Length (um):") -> (index of element=w931:i32)  [unwired: 1 in]
                n547 = Equal?(x=w931, y=-1) -> (x = y?=w930:bool)
                n548 = case shown="False" w930 {
                  tunnel: w921 -> [w941 w944]
                  tunnel: w931 -> [w938 _]
                  tunnel: [w937 w944] -> w929
                  frame False {
                    n549 = local read "New: Length"() -> (w934:dbl)
                    n550 = Divide(x=w938, y=3) -> (x/y=w940:dbl)
                    n551 = Format Value(format string="%#g", value (0)=w934) -> (output string=w935:string)  [unwired: 1 in]
                    n552 = To Word Integer(number=w940) -> (16bit integer=w939:i16)
                    n553 = Replace Array Subset(array=w941, new element=w935, index (row)=w939, index (col)=1) -> (w937:string[][])
                  }
                  frame True {
                  }
                }
                n554 = local write "Save Array"(w929) -> ()
              }
              frame #3 {
                n555 = local read "Save Array"() -> (w946:string[][])
                n556 = Array Size(array=w946) -> (size(s)=w951:i32[])
                n557 = Array Subset(array=w946, index (row)=0, index (col)=0, length (col)=3) -> (w947:string[][])  [unwired: 1 in]
                n558 = Index Array(array=w951, index=0) -> (element=w953:i32)
                n559 = Reshape Array(w947, w953) -> (w945:string[])
                n560 = Search 1D Array(1D array=w945, element="Width (um):") -> (index of element=w956:i32)  [unwired: 1 in]
                n561 = Equal?(x=w956, y=-1) -> (x = y?=w955:bool)
                n562 = case shown="False" w955 {
                  tunnel: w956 -> [w964 _]
                  tunnel: w946 -> [w963 w969]
                  tunnel: [w962 w969] -> w954
                  frame False {
                    n563 = local read "New: Width"() -> (w959:dbl)
                    n564 = Divide(x=w964, y=3) -> (x/y=w966:dbl)
                    n565 = To Word Integer(number=w966) -> (16bit integer=w965:i16)
                    n566 = Format Value(format string="%#g", value (0)=w959) -> (output string=w960:string)  [unwired: 1 in]
                    n567 = Replace Array Subset(array=w963, new element=w960, index (row)=w965, index (col)=1) -> (w962:string[][])
                  }
                  frame True {
                  }
                }
                n568 = local write "Save Array"(w954) -> ()
              }
              frame #4 {
                w979 = "Sample Temp (K):"
                n569 = local read "Save Array"() -> (w971:string[][])
                n570 = Array Size(array=w971) -> (size(s)=w976:i32[])
                n571 = Array Subset(array=w971, index (row)=0, index (col)=0, length (col)=3) -> (w972:string[][])  [unwired: 1 in]
                n572 = Index Array(array=w976, index=0) -> (element=w978:i32)
                n573 = Reshape Array(w972, w978) -> (w970:string[])
                n574 = Search 1D Array(1D array=w970, element=w979) -> (index of element=w982:i32)  [unwired: 1 in]
                n575 = Equal?(x=w982, y=-1) -> (x = y?=w981:bool)
                n576 = case shown="True" w981 {
                  tunnel: w971 -> [w991 w1005]
                  tunnel: w982 -> [w988 _]
                  tunnel: [w987 w1004] -> w980
                  tunnel: w970 -> [_ w1007]
                  tunnel: w979 -> [_ w994]
                  frame False {
                    n577 = local read "New: Temp"() -> (w985:dbl)
                    n578 = Divide(x=w988, y=3) -> (x/y=w990:dbl)
                    n579 = Format Value(format string="%#g", value (0)=w985) -> (output string=w984:string)  [unwired: 1 in]
                    n580 = To Word Integer(number=w990) -> (16bit integer=w989:i16)
                    n581 = Replace Array Subset(array=w991, new element=w984, index (row)=w989, index (col)=1) -> (w987:string[][])
                  }
                  frame True {
                    n582 = local read "New: Temp"() -> (w996:dbl)
                    n583 = Search 1D Array(1D array=w1007, element="Width (um):") -> (index of element=w1001:i32)  [unwired: 1 in]
                    n584 = Divide(x=w1001, y=3) -> (x/y=w1002:dbl)
                    n585 = To Word Integer(number=w1002) -> (16bit integer=w1000:i16)
                    n586 = Format Value(format string="%#g", value (0)=w996) -> (output string=w995:string)  [unwired: 1 in]
                    n587 = Build Array(w994, w995) -> (w998:string[])
                    n588 = Increment(x=w1000) -> (x+1=w999:i16)
                    n589 = Insert Into Array(array=w1005, index (row)=w999, new element=w998) -> (w1004:string[][])  [unwired: 1 in]
                  }
                }
                n590 = local write "Save Array"(w980) -> ()
              }
              frame #5 {
                w1017 = "Mobility-Sat (cm^2/Vs):"
                n591 = local read "Save Array"() -> (w1009:string[][])
                n592 = Array Size(array=w1009) -> (size(s)=w1014:i32[])
                n593 = Array Subset(array=w1009, index (row)=0, index (col)=0, length (col)=3) -> (w1010:string[][])  [unwired: 1 in]
                n594 = Index Array(array=w1014, index=0) -> (element=w1016:i32)
                n595 = Reshape Array(w1010, w1016) -> (w1008:string[])
                n596 = Search 1D Array(1D array=w1008, element=w1017) -> (index of element=w1020:i32)  [unwired: 1 in]
                n597 = Equal?(x=w1020, y=-1) -> (x = y?=w1019:bool)
                n598 = case shown="True" w1019 {
                  tunnel: w1009 -> [w1030 w1040]
                  tunnel: w1020 -> [w1027 _]
                  tunnel: [w1026 w1039] -> w1018
                  tunnel: w1008 -> [_ w1037]
                  tunnel: w1017 -> [_ w1035]
                  frame False {
                    n599 = local read "Re-Calculated Values Cluster"() -> (w1023:T10)
                    n600 = Unbundle By Name(w1023) -> ("Mobility-Sat"=w1022:dbl)
                    n601 = Divide(x=w1027, y=3) -> (x/y=w1029:dbl)
                    n602 = To Word Integer(number=w1029) -> (16bit integer=w1028:i16)
                    n603 = Format Value(format string="%#g", value (0)=w1022) -> (output string=w1024:string)  [unwired: 1 in]
                    n604 = Replace Array Subset(array=w1030, new element=w1024, index (row)=w1028, index (col)=1) -> (w1026:string[][])
                  }
                  frame True {
                    n605 = local read "Re-Calculated Values Cluster"() -> (w1034:T10)
                    n606 = Unbundle By Name(w1034) -> ("Mobility-Sat"=w1033:dbl)
                    n607 = Search 1D Array(1D array=w1037, element="Mobility (cm^2/Vs):") -> (index of element=w1043:i32)  [unwired: 1 in]
                    n608 = Divide(x=w1043, y=3) -> (x/y=w1044:dbl)
                    n609 = To Word Integer(number=w1044) -> (16bit integer=w1036:i16)
                    n610 = Format Value(format string="%#g", value (0)=w1033) -> (output string=w1038:string)  [unwired: 1 in]
                    n611 = Build Array(w1035, w1038) -> (w1042:string[])
                    n612 = Replace Array Subset(array=w1040, new element=w1042, index (row)=w1036) -> (w1039:string[][])  [unwired: 1 in]
                  }
                }
                n613 = local write "Save Array"(w1018) -> ()
              }
              frame #6 {
                w1056 = "Mobility-Lin (cm^2/Vs):"
                n614 = local read "Save Array"() -> (w1047:string[][])
                n615 = Array Size(array=w1047) -> (size(s)=w1053:i32[])
                n616 = Array Subset(array=w1047, index (row)=0, index (col)=0, length (col)=3) -> (w1049:string[][])  [unwired: 1 in]
                n617 = Index Array(array=w1053, index=0) -> (element=w1055:i32)
                n618 = Reshape Array(w1049, w1055) -> (w1048:string[])
                n619 = Search 1D Array(1D array=w1048, element=w1056) -> (index of element=w1059:i32)  [unwired: 1 in]
                n620 = Equal?(x=w1059, y=-1) -> (x = y?=w1058:bool)
                n621 = case shown="True" w1058 {
                  tunnel: w1047 -> [w1069 w1077]
                  tunnel: w1059 -> [w1066 _]
                  tunnel: [w1065 w1076] -> w1057
                  tunnel: w1048 -> [_ w1075]
                  tunnel: w1056 -> [_ w1074]
                  frame False {
                    n622 = local read "Re-Calculated Values Cluster"() -> (w1062:T10)
                    n623 = Unbundle By Name(w1062) -> ("Moblitity-Lin"=w1061:dbl)
                    n624 = Divide(x=w1066, y=3) -> (x/y=w1068:dbl)
                    n625 = To Word Integer(number=w1068) -> (16bit integer=w1067:i16)
                    n626 = Format Value(format string="%#g", value (0)=w1061) -> (output string=w1063:string)  [unwired: 1 in]
                    n627 = Replace Array Subset(array=w1069, new element=w1063, index (row)=w1067, index (col)=1) -> (w1065:string[][])
                  }
                  frame True {
                    n628 = local read "Re-Calculated Values Cluster"() -> (w1073:T10)
                    n629 = Unbundle By Name(w1073) -> ("Moblitity-Lin"=w1072:dbl)
                    n630 = Search 1D Array(1D array=w1075, element="Mobility-Sat (cm^2/Vs):") -> (index of element=w1082:i32)  [unwired: 1 in]
                    n631 = Divide(x=w1082, y=3) -> (x/y=w1083:dbl)
                    n632 = To Word Integer(number=w1083) -> (16bit integer=w1081:i16)
                    n633 = Format Value(format string="%#g", value (0)=w1072) -> (output string=w1086:string)  [unwired: 1 in]
                    n634 = Build Array(w1074, w1086) -> (w1079:string[])
                    n635 = Increment(x=w1081) -> (x+1=w1080:i16)
                    n636 = Insert Into Array(array=w1077, index (row)=w1080, new element=w1079) -> (w1076:string[][])  [unwired: 1 in]
                  }
                }
                n637 = local write "Save Array"(w1057) -> ()
              }
              frame #7 {
                w1096 = "On/Off I-Sat:"
                n638 = local read "Save Array"() -> (w1087:string[][])
                n639 = Array Size(array=w1087) -> (size(s)=w1093:i32[])
                n640 = Array Subset(array=w1087, index (row)=0, index (col)=0, length (col)=3) -> (w1089:string[][])  [unwired: 1 in]
                n641 = Index Array(array=w1093, index=0) -> (element=w1095:i32)
                n642 = Reshape Array(w1089, w1095) -> (w1088:string[])
                n643 = Search 1D Array(1D array=w1088, element=w1096) -> (index of element=w1099:i32)  [unwired: 1 in]
                n644 = Equal?(x=w1099, y=-1) -> (x = y?=w1098:bool)
                n645 = case shown="True" w1098 {
                  tunnel: w1087 -> [w1109 w1118]
                  tunnel: w1099 -> [w1106 _]
                  tunnel: [w1105 w1119] -> w1097
                  tunnel: w1088 -> [_ w1116]
                  tunnel: w1096 -> [_ w1114]
                  frame False {
                    n646 = local read "Calculated Values Cluster"() -> (w1102:T10)
                    n647 = Divide(x=w1106, y=3) -> (x/y=w1108:dbl)
                    n648 = Unbundle By Name(w1102) -> ("On/Off"=w1101:dbl)
                    n649 = To Word Integer(number=w1108) -> (16bit integer=w1107:i16)
                    n650 = Format Value(format string="%#g", value (0)=w1101) -> (output string=w1103:string)  [unwired: 1 in]
                    n651 = Replace Array Subset(array=w1109, new element=w1103, index (row)=w1107, index (col)=1) -> (w1105:string[][])
                  }
                  frame True {
                    n652 = local read "Calculated Values Cluster"() -> (w1113:T10)
                    n653 = Unbundle By Name(w1113) -> ("On/Off"=w1112:dbl)
                    n654 = Search 1D Array(1D array=w1116, element="On/Off Current:") -> (index of element=w1122:i32)  [unwired: 1 in]
                    n655 = Divide(x=w1122, y=3) -> (x/y=w1123:dbl)
                    n656 = To Word Integer(number=w1123) -> (16bit integer=w1115:i16)
                    n657 = Format Value(format string="%#g", value (0)=w1112) -> (output string=w1117:string)  [unwired: 1 in]
                    n658 = Build Array(w1114, w1117) -> (w1121:string[])
                    n659 = Replace Array Subset(array=w1118, new element=w1121, index (row)=w1115) -> (w1119:string[][])  [unwired: 1 in]
                  }
                }
                n660 = local write "Save Array"(w1097) -> ()
              }
              frame #8 {
                w1135 = "Off I-Sat (A):"
                n661 = local read "Save Array"() -> (w1126:string[][])
                n662 = Array Size(array=w1126) -> (size(s)=w1132:i32[])
                n663 = Array Subset(array=w1126, index (row)=0, index (col)=0, length (col)=3) -> (w1128:string[][])  [unwired: 1 in]
                n664 = Index Array(array=w1132, index=0) -> (element=w1134:i32)
                n665 = Reshape Array(w1128, w1134) -> (w1127:string[])
                n666 = Search 1D Array(1D array=w1127, element=w1135) -> (index of element=w1138:i32)  [unwired: 1 in]
                n667 = Equal?(x=w1138, y=-1) -> (x = y?=w1137:bool)
                n668 = case shown="True" w1137 {
                  tunnel: w1126 -> [w1148 w1156]
                  tunnel: w1138 -> [w1145 _]
                  tunnel: [w1144 w1155] -> w1136
                  tunnel: w1127 -> [_ w1154]
                  tunnel: w1135 -> [_ w1153]
                  frame False {
                    # "New Data File"
                    n669 = local read "Calculated Values Cluster"() -> (w1141:T10)
                    n670 = Unbundle By Name(w1141) -> ("Off Current"=w1140:dbl)
                    n671 = Divide(x=w1145, y=3) -> (x/y=w1147:dbl)
                    n672 = Format Value(format string="%#g", value (0)=w1140) -> (output string=w1142:string)  [unwired: 1 in]
                    n673 = To Word Integer(number=w1147) -> (16bit integer=w1146:i16)
                    n674 = Replace Array Subset(array=w1148, new element=w1142, index (row)=w1146, index (col)=1) -> (w1144:string[][])
                  }
                  frame True {
                    # "Old Data File"
                    n675 = local read "Calculated Values Cluster"() -> (w1152:T10)
                    n676 = Unbundle By Name(w1152) -> ("Off Current"=w1151:dbl)
                    n677 = Search 1D Array(1D array=w1154, element="On/Off I-Sat:") -> (index of element=w1161:i32)  [unwired: 1 in]
                    n678 = Divide(x=w1161, y=3) -> (x/y=w1162:dbl)
                    n679 = To Word Integer(number=w1162) -> (16bit integer=w1160:i16)
                    n680 = Format Value(format string="%#g", value (0)=w1151) -> (output string=w1165:string)  [unwired: 1 in]
                    n681 = Build Array(w1153, w1165) -> (w1158:string[])
                    n682 = Increment(x=w1160) -> (x+1=w1159:i16)
                    n683 = Insert Into Array(array=w1156, index (row)=w1159, new element=w1158) -> (w1155:string[][])  [unwired: 1 in]
                  }
                }
                n684 = local write "Save Array"(w1136) -> ()
              }
              frame #9 {
                w1167 = "Vt-Sat (V):"
                n685 = local read "Save Array"() -> (w1168:string[][])
                n686 = Array Size(array=w1168) -> (size(s)=w1173:i32[])
                n687 = Array Subset(array=w1168, index (row)=0, index (col)=0, length (col)=3) -> (w1169:string[][])  [unwired: 1 in]
                n688 = Index Array(array=w1173, index=0) -> (element=w1175:i32)
                n689 = Reshape Array(w1169, w1175) -> (w1166:string[])
                n690 = Search 1D Array(1D array=w1166, element=w1167) -> (index of element=w1178:i32)  [unwired: 1 in]
                n691 = Equal?(x=w1178, y=-1) -> (x = y?=w1177:bool)
                n692 = case shown="True" w1177 {
                  tunnel: w1168 -> [w1187 w1197]
                  tunnel: w1178 -> [w1183 _]
                  tunnel: [w1182 w1196] -> w1176
                  tunnel: w1167 -> [_ w1195]
                  tunnel: w1166 -> [_ w1194]
                  frame False {
                    n693 = local read "Re-Calculated Values Cluster"() -> (w1181:T10)
                    n694 = Unbundle By Name(w1181) -> ("Vt-Sat"=w1180:dbl)
                    n695 = Divide(x=w1183, y=3) -> (x/y=w1186:dbl)
                    n696 = To Word Integer(number=w1186) -> (16bit integer=w1185:i16)
                    n697 = Number To Fractional String(number=w1180) -> (F-format string=w1184:string)  [unwired: 3 in]
                    n698 = Replace Array Subset(array=w1187, new element=w1184, index (row)=w1185, index (col)=1) -> (w1182:string[][])
                  }
                  frame True {
                    n699 = local read "Re-Calculated Values Cluster"() -> (w1191:T10)
                    n700 = Unbundle By Name(w1191) -> ("Vt-Sat"=w1190:dbl)
                    n701 = Search 1D Array(1D array=w1194, element="Threshold V (V):") -> (index of element=w1193:i32)  [unwired: 1 in]
                    n702 = Divide(x=w1193, y=3) -> (x/y=w1200:dbl)
                    n703 = To Word Integer(number=w1200) -> (16bit integer=w1192:i16)
                    n704 = Format Value(format string="%#g", value (0)=w1190) -> (output string=w1203:string)  [unwired: 1 in]
                    n705 = Build Array(w1195, w1203) -> (w1199:string[])
                    n706 = Replace Array Subset(array=w1197, new element=w1199, index (row)=w1192) -> (w1196:string[][])  [unwired: 1 in]
                  }
                }
                n707 = local write "Save Array"(w1176) -> ()
              }
              frame #10 {
                n708 = disable-structure shown="Disabled" {
                  frame Disabled {
                    n709 = local read "Save Array"() -> (w1204:string[][])
                    n710 = Array Size(array=w1204) -> (size(s)=w1210:i32[])
                    n711 = Array Subset(array=w1204, index (row)=0, index (col)=0, length (col)=3) -> (w1206:string[][])  [unwired: 1 in]
                    n712 = Index Array(array=w1210, index=0) -> (element=w1212:i32)
                    n713 = Reshape Array(w1206, w1212) -> (w1205:string[])
                    n714 = Search 1D Array(1D array=w1205, element="VT-Lin (V):") -> (index of element=w1215:i32)  [unwired: 1 in]
                    n715 = Equal?(x=w1215, y=-1) -> (x = y?=w1214:bool)
                    n716 = case shown="False" w1214 {
                      tunnel: w1204 -> [w1224 w1227]
                      tunnel: w1215 -> [w1221 _]
                      tunnel: [w1220 w1227] -> w1213
                      frame False {
                        n717 = Divide(x=w1221, y=3) -> (x/y=w1223:dbl)
                        n718 = To Word Integer(number=w1223) -> (16bit integer=w1222:i16)
                        n719 = Format Value(format string="%#g") -> (output string=w1218:string)  [unwired: 2 in]
                        n720 = Replace Array Subset(array=w1224, new element=w1218, index (row)=w1222, index (col)=1) -> (w1220:string[][])
                      }
                      frame True {
                      }
                    }
                    n721 = local write "Save Array"(w1213) -> ()
                  }
                  frame Enabled {
                  }
                }
              }
              frame #11 {
                w1228 = "STS-Sat (V/decade):"
                n722 = local read "Save Array"() -> (w1230:string[][])
                n723 = Array Size(array=w1230) -> (size(s)=w1235:i32[])
                n724 = Array Subset(array=w1230, index (row)=0, index (col)=0, length (col)=3) -> (w1231:string[][])  [unwired: 1 in]
                n725 = Index Array(array=w1235, index=0) -> (element=w1237:i32)
                n726 = Reshape Array(w1231, w1237) -> (w1229:string[])
                n727 = Search 1D Array(1D array=w1229, element=w1228) -> (index of element=w1240:i32)  [unwired: 1 in]
                n728 = Equal?(x=w1240, y=-1) -> (x = y?=w1239:bool)
                n729 = case shown="True" w1239 {
                  tunnel: w1230 -> [w1250 w1258]
                  tunnel: w1240 -> [w1247 _]
                  tunnel: [w1246 w1259] -> w1238
                  tunnel: w1229 -> [_ w1257]
                  tunnel: w1228 -> [_ w1256]
                  frame False {
                    # "Current Data File"
                    n730 = local read "Re-Calculated Values Cluster"() -> (w1242:T10)
                    n731 = Unbundle By Name(w1242) -> ("STS"=w1243:dbl)
                    n732 = Divide(x=w1247, y=3) -> (x/y=w1249:dbl)
                    n733 = To Word Integer(number=w1249) -> (16bit integer=w1248:i16)
                    n734 = Format Value(format string="%#g", value (0)=w1243) -> (output string=w1244:string)  [unwired: 1 in]
                    n735 = Replace Array Subset(array=w1250, new element=w1244, index (row)=w1248, index (col)=1) -> (w1246:string[][])
                  }
                  frame True {
                    # "Old Data File"
                    n736 = local read "Re-Calculated Values Cluster"() -> (w1253:T10)
                    n737 = Unbundle By Name(w1253) -> ("STS"=w1254:dbl)
                    n738 = Search 1D Array(1D array=w1257, element="S.T.S. (V/decade):") -> (index of element=w1262:i32)  [unwired: 1 in]
                    n739 = Divide(x=w1262, y=3) -> (x/y=w1263:dbl)
                    n740 = To Word Integer(number=w1263) -> (16bit integer=w1255:i16)
                    n741 = Format Value(format string="%#g", value (0)=w1254) -> (output string=w1266:string)  [unwired: 1 in]
                    n742 = Build Array(w1256, w1266) -> (w1261:string[])
                    n743 = Replace Array Subset(array=w1258, new element=w1261, index (row)=w1255) -> (w1259:string[][])  [unwired: 1 in]
                  }
                }
                n744 = local write "Save Array"(w1238) -> ()
              }
              frame #12 {
                w1267 = "Trap Density-VT (Traps/Vcm^2):"
                n745 = local read "Save Array"() -> (w1269:string[][])
                n746 = Array Size(array=w1269) -> (size(s)=w1274:i32[])
                n747 = Array Subset(array=w1269, index (row)=0, index (col)=0, length (col)=3) -> (w1270:string[][])  [unwired: 1 in]
                n748 = Index Array(array=w1274, index=0) -> (element=w1276:i32)
                n749 = Reshape Array(w1270, w1276) -> (w1268:string[])
                n750 = Search 1D Array(1D array=w1268, element=w1267) -> (index of element=w1279:i32)  [unwired: 1 in]
                n751 = Equal?(x=w1279, y=-1) -> (x = y?=w1278:bool)
                n752 = case shown="True" w1278 {
                  tunnel: w1269 -> [w1289 w1296]
                  tunnel: w1279 -> [w1285 _]
                  tunnel: [w1284 w1297] -> w1277
                  tunnel: w1268 -> [_ w1295]
                  tunnel: w1267 -> [_ w1294]
                  frame False {
                    n753 = local read "Re-Calculated Values Cluster"() -> (w1282:T10)
                    n754 = Unbundle By Name(w1282) -> ("Trap Density-VT"=w1281:dbl)
                    n755 = Divide(x=w1285, y=3) -> (x/y=w1288:dbl)
                    n756 = To Word Integer(number=w1288) -> (16bit integer=w1287:i16)
                    n757 = Format Value(format string="%#g", value (0)=w1281) -> (output string=w1286:string)  [unwired: 1 in]
                    n758 = Replace Array Subset(array=w1289, new element=w1286, index (row)=w1287, index (col)=1) -> (w1284:string[][])
                  }
                  frame True {
                    n759 = local read "Re-Calculated Values Cluster"() -> (w1293:T10)
                    n760 = Unbundle By Name(w1293) -> ("Trap Density-VT"=w1292:dbl)
                    n761 = Search 1D Array(1D array=w1295, element="STS-Sat (V/decade):") -> (index of element=w1302:i32)  [unwired: 1 in]
                    n762 = Divide(x=w1302, y=3) -> (x/y=w1301:dbl)
                    n763 = To Word Integer(number=w1301) -> (16bit integer=w1303:i16)
                    n764 = Format Value(format string="%#g", value (0)=w1292) -> (output string=w1298:string)  [unwired: 1 in]
                    n765 = Build Array(w1294, w1298) -> (w1305:string[])
                    n766 = Increment(x=w1303) -> (x+1=w1304:i16)
                    n767 = Insert Into Array(array=w1296, index (row)=w1304, new element=w1305) -> (w1297:string[][])  [unwired: 1 in]
                  }
                }
                n768 = local write "Save Array"(w1277) -> ()
              }
              frame #13 {
                w1307 = "Trap Density-STS (Traps/Vcm^2):"
                n769 = local read "Save Array"() -> (w1309:string[][])
                n770 = Array Size(array=w1309) -> (size(s)=w1314:i32[])
                n771 = Array Subset(array=w1309, index (row)=0, index (col)=0, length (col)=3) -> (w1310:string[][])  [unwired: 1 in]
                n772 = Index Array(array=w1314, index=0) -> (element=w1316:i32)
                n773 = Reshape Array(w1310, w1316) -> (w1308:string[])
                n774 = Search 1D Array(1D array=w1308, element=w1307) -> (index of element=w1319:i32)  [unwired: 1 in]
                n775 = Equal?(x=w1319, y=-1) -> (x = y?=w1318:bool)
                n776 = case shown="True" w1318 {
                  tunnel: w1309 -> [w1329 w1336]
                  tunnel: w1319 -> [w1326 _]
                  tunnel: [w1325 w1337] -> w1317
                  tunnel: w1308 -> [_ w1335]
                  tunnel: w1307 -> [_ w1334]
                  frame False {
                    n777 = local read "Re-Calculated Values Cluster"() -> (w1322:T10)
                    n778 = Unbundle By Name(w1322) -> ("Trap Density-STS"=w1321:dbl)
                    n779 = Divide(x=w1326, y=3) -> (x/y=w1328:dbl)
                    n780 = To Word Integer(number=w1328) -> (16bit integer=w1327:i16)
                    n781 = Format Value(format string="%#g", value (0)=w1321) -> (output string=w1323:string)  [unwired: 1 in]
                    n782 = Replace Array Subset(array=w1329, new element=w1323, index (row)=w1327, index (col)=1) -> (w1325:string[][])
                  }
                  frame True {
                    n783 = local read "Re-Calculated Values Cluster"() -> (w1333:T10)
                    n784 = Unbundle By Name(w1333) -> ("Trap Density-STS"=w1332:dbl)
                    n785 = Search 1D Array(1D array=w1335, element="Trap Density-VT (Traps/Vcm^2):") -> (index of element=w1342:i32)  [unwired: 1 in]
                    n786 = Divide(x=w1342, y=3) -> (x/y=w1343:dbl)
                    n787 = To Word Integer(number=w1343) -> (16bit integer=w1341:i16)
                    n788 = Format Value(format string="%#g", value (0)=w1332) -> (output string=w1346:string)  [unwired: 1 in]
                    n789 = Build Array(w1334, w1346) -> (w1339:string[])
                    n790 = Increment(x=w1341) -> (x+1=w1340:i16)
                    n791 = Insert Into Array(array=w1336, index (row)=w1340, new element=w1339) -> (w1337:string[][])  [unwired: 1 in]
                  }
                }
                n792 = local write "Save Array"(w1317) -> ()
              }
            }
            n793 = local read "New: Temp"() -> (w854:dbl)
            n794 = local read "New: Width"() -> (w855:dbl)
            n795 = local read "New: Length"() -> (w857:dbl)
            n796 = local read "Index"() -> (w856:string)
            n797 = To Single Precision Float(number=w854) -> (single precision float=w871:sgl)
            n798 = Number To Decimal String(number=w871) -> (decimal integer string=w866:string)  [unwired: 1 in]
            n799 = To Single Precision Float(number=w855) -> (single precision float=w870:sgl)
            n800 = To Single Precision Float(number=w857) -> (single precision float=w869:sgl)
            n801 = Strip Path(path=w853) -> (stripped path=w858:path)  [unwired: 1 out]
            n802 = Number To Decimal String(number=w869) -> (decimal integer string=w864:string)  [unwired: 1 in]
            n803 = Number To Decimal String(number=w870) -> (decimal integer string=w863:string)  [unwired: 1 in]
            n804 = Concatenate Strings("_", w866, "K") -> (w868:string)
            n805 = call "Build Text"("Temp"=w868, "Index"=w856, "Length"=w864, "Width"=w863) -> ("Result"=w862:string)  [unwired: 10 in, 1 out]
            n806 = Path To String(path=w858) -> (string=w860:string)
            n807 = Concatenate Strings(w860, "\\", w862) -> (w861:string)
            n808 = String To Path(string=w861) -> (path=w852:path)
          }
          frame #1 {
            n809 = flat-sequence {
              tunnel: w1350 -> [w1352]
              tunnel: w1349 -> [w1351]
              tunnel: [w1351] -> w1348
              tunnel: w1348 -> [w1358]
              tunnel: w1347 -> [w1357]
              frame #0 {
                n810 = Equal?(x=w1352, y=w1351) -> (x = y?=w1353:bool)
                n811 = case shown="False" w1353 {
                  tunnel: w1352 -> [w1356 _]
                  tunnel: w1351 -> [w1355 _]
                  frame False {
                    n812 = Move(source path=w1356, 9:TRUE, 10:w1355) -> ()  [unwired: 2 in, 3 out]
                  }
                  frame True {
                  }
                }
              }
              frame #1 {
                n813 = local write "Transfer File"(w1358) -> ()
                n814 = call-poly <vilib>:"Write To Spreadsheet File.vi"("2D data"=w1357, "file path (dialog if empty)"=w1358) -> ()  [unwired: 6 in, 1 out]
              }
            }
          }
        }
        n815 = Unbundle By Name(w838) -> ("Save Next"=w837:bool)
        n816 = Cluster To Array(cluster=w843) -> (array=w842:bool[])
        n817 = Boolean Array To Number(Boolean array=w842) -> (number=w841:u32)
        n818 = Equal To 0?(x=w841) -> (x = 0?=w840:bool)
        n819 = case shown="True" w840 {
          tunnel: [MegaAwesome_States."Read Data" w850] -> w839
          tunnel: w837 -> [_ w847]
          frame False {
          }
          frame True {
            n820 = Select(t=MegaAwesome_States."No Event", s=w847, f=MegaAwesome_States."Next File") -> (s? t:f=w850:T3)
          }
        }
      }
      frame "Exit" {
        n821 = flat-sequence {
          tunnel: [w1369] -> w1360
          tunnel: [w1369] -> w1359
          frame #0 {
            w1368 = FALSE
            n822 = property on="Next File" class="Bool (strict)"("Value"=w1368) -> (error out=w1363:errorcluster)  [unwired: 2 in, 1 out]
            n823 = property on="Previous File" class="Bool (strict)"(error in=w1363, "Value"=w1368) -> (error out=w1364:errorcluster)  [unwired: 1 in, 1 out]
            n824 = property on="Save" class="Bool (strict)"(error in=w1364, "Value"=w1368) -> (error out=w1365:errorcluster)  [unwired: 1 in, 1 out]
            n825 = property on="Export" class="Bool (strict)"("Value"=w1368) -> ()  [unwired: 2 in, 2 out]
            n826 = property on="Save Next" class="Bool (strict)"(error in=w1365, "Value"=w1368) -> (error out=w1366:errorcluster)  [unwired: 1 in, 1 out]
            n827 = property on="Discard" class="Bool (strict)"(error in=w1366, "Value"=w1368) -> (error out=w1367:errorcluster)  [unwired: 1 in, 1 out]
            n828 = property on="Save Lines" class="Bool (strict)"(error in=w1367, "Value"=w1368) -> ()  [unwired: 1 in, 2 out]
            n829 = property on="Close" class="Bool (strict)"("Value"=w1368) -> ()  [unwired: 2 in, 2 out]
            n830 = property on="Disable Flag" class="Bool (strict)"("Value"=w1368) -> ()  [unwired: 2 in, 2 out]
            n831 = call "IMAQ Dispose"("All Images? (No)"=TRUE) -> ()  [unwired: 5 in, 1 out]
          }
          frame #1 {
            w1369 = MegaAwesome_States."Exit"
          }
        }
      }
      frame "Save Lines" {
        n832 = Build Path(base path=w1371, name or relative path="ROI") -> (appended path=w1374:path)
        n833 = call <vilib>:"Check if File or Folder Exists.vi"("path"=w1374) -> ("file or folder exists?"=w1372:bool, "dup path"=w1375:path)  [unwired: 8 in, 1 out]
        n834 = case shown="False" w1372 {
          tunnel: w1375 -> [w1383 w1384]
          tunnel: [w1382 w1384] -> w1379
          frame False {
            n835 = Create Folder(path (use dialog)=w1383) -> (created path=w1382:path)  [unwired: 2 in, 2 out]
          }
          frame True {
          }
        }
        n836 = local read "Index"() -> (w1370:string)
        n837 = property on="Image Out" class="ImageControl"() -> ("ROI"=w1376:T13)  [unwired: 2 in, 2 out]
        n838 = Build Path(base path=w1379, name or relative path=w1370) -> (appended path=w1378:path)
        n839 = Flatten To String(anything=w1376) -> (data string=w1377:string)  [unwired: 3 in, 2 out]
        n840 = Write to Text File(file (use dialog)=w1378, text=w1377) -> ()  [unwired: 2 in, 3 out]
      }
      frame "Export" {
        n841 = flat-sequence {
          tunnel: w1385 -> [w1438]
          frame #0 {
            n842 = stacked-sequence {
              frame #0 {
                n843 = local read "Independant Variable:"() -> (w1388:string)
                n844 = Equal?(x=w1388, y="Length (um):") -> (x = y?=w1389:bool)
                n845 = case shown="True" w1389 {
                  frame False {
                  }
                  frame True {
                    n846 = local write "X Axis Display Type"("1") -> ()
                    n847 = local write "Opj X Axis"("2") -> ()
                  }
                }
              }
              frame #1 {
                n848 = local read "Independant Variable:"() -> (w1393:string)
                n849 = Equal?(x=w1393, y="Sample Temp (K):") -> (x = y?=w1394:bool)
                n850 = case shown="True" w1394 {
                  frame False {
                  }
                  frame True {
                    n851 = local write "X Axis Display Type"("1") -> ()
                    n852 = local write "Opj X Axis"("1") -> ()
                  }
                }
              }
              frame #2 {
                n853 = local read "Independant Variable:"() -> (w1398:string)
                n854 = Equal?(x=w1398, y="Mobility-Sat (cm^2/Vs):") -> (x = y?=w1399:bool)
                n855 = case shown="True" w1399 {
                  frame False {
                  }
                  frame True {
                    n856 = local write "X Axis Display Type"("2") -> ()
                    n857 = local write "Opj X Axis"("2") -> ()
                  }
                }
              }
              frame #3 {
                n858 = local read "Independant Variable:"() -> (w1403:string)
                n859 = Equal?(x=w1403, y="Mobility-Lin (cm^2/Vs):") -> (x = y?=w1404:bool)
                n860 = case shown="True" w1404 {
                  frame False {
                  }
                  frame True {
                    n861 = local write "X Axis Display Type"("2") -> ()
                    n862 = local write "Opj X Axis"("2") -> ()
                  }
                }
              }
              frame #4 {
                n863 = local read "Independant Variable:"() -> (w1408:string)
                n864 = Equal?(x=w1408, y="On/Off I-Sat:") -> (x = y?=w1409:bool)
                n865 = case shown="True" w1409 {
                  frame False {
                  }
                  frame True {
                    n866 = local write "X Axis Display Type"("2") -> ()
                    n867 = local write "Opj X Axis"("2") -> ()
                  }
                }
              }
              frame #5 {
                n868 = local read "Independant Variable:"() -> (w1413:string)
                n869 = Equal?(x=w1413, y="Off I-Sat (A):") -> (x = y?=w1414:bool)
                n870 = case shown="True" w1414 {
                  frame False {
                  }
                  frame True {
                    n871 = local write "X Axis Display Type"("2") -> ()
                    n872 = local write "Opj X Axis"("2") -> ()
                  }
                }
              }
              frame #6 {
                n873 = local read "Independant Variable:"() -> (w1418:string)
                n874 = Equal?(x=w1418, y="Vt-Sat (V):") -> (x = y?=w1419:bool)
                n875 = case shown="True" w1419 {
                  frame False {
                  }
                  frame True {
                    n876 = local write "X Axis Display Type"("1") -> ()
                    n877 = local write "Opj X Axis"("1") -> ()
                  }
                }
              }
              frame #7 {
                n878 = local read "Independant Variable:"() -> (w1423:string)
                n879 = Equal?(x=w1423, y="STS-Sat (V/decade):") -> (x = y?=w1424:bool)
                n880 = case shown="True" w1424 {
                  frame False {
                  }
                  frame True {
                    n881 = local write "X Axis Display Type"("1") -> ()
                    n882 = local write "Opj X Axis"("1") -> ()
                  }
                }
              }
              frame #8 {
                n883 = local read "Independant Variable:"() -> (w1428:string)
                n884 = Equal?(x=w1428, y="Trap Density-VT (Traps/Vcm^2):") -> (x = y?=w1429:bool)
                n885 = case shown="True" w1429 {
                  frame False {
                  }
                  frame True {
                    n886 = local write "X Axis Display Type"("2") -> ()
                    n887 = local write "Opj X Axis"("2") -> ()
                  }
                }
              }
              frame #9 {
                n888 = local read "Independant Variable:"() -> (w1433:string)
                n889 = Equal?(x=w1433, y="Trap Density-STS (Traps/Vcm^2):") -> (x = y?=w1434:bool)
                n890 = case shown="True" w1434 {
                  frame False {
                  }
                  frame True {
                    n891 = local write "X Axis Display Type"("2") -> ()
                    n892 = local write "Opj X Axis"("2") -> ()
                  }
                }
              }
            }
          }
          frame #1 {
            n893 = local read "Transfer Folder"() -> (w1443:path)
            n894 = Build Path(base path=w1443, name or relative path="Stats") -> (appended path=w1444:path)
            n895 = call <vilib>:"Check if File or Folder Exists.vi"("path"=w1444) -> ("file or folder exists?"=w1458:bool, "dup path"=w1457:path)  [unwired: 8 in, 1 out]
            n896 = call <userlib>:"OA_ConnectToOrigin.vi"() -> ("error out"=w1455:errorcluster, "Origin.IOApplication"=w1456:refnum<k7>)  [unwired: 8 in]
            n897 = case shown="False" w1458 {
              tunnel: w1457 -> [w1631 w1632]
              tunnel: [w1630 w1632] -> w1442
              frame False {
                n898 = Create Folder(path (use dialog)=w1631) -> (created path=w1630:path)  [unwired: 2 in, 2 out]
              }
              frame True {
              }
            }
            n899 = call "File Dialog"("start path"=w1444) -> ("selected path"=w1446:path)  [unwired: 11 in, 3 out]
            n900 = call <userlib>:"OA_Load.vi"("error in (no error)"=w1455, "Path"=w1438, "Origin.IOApplication"=w1456) -> ("error out"=w1453:errorcluster, "Origin.IOApplication"=w1454:refnum<k7>)  [unwired: 1 out]
            n901 = call "OAExecute.vi"("script"="document -m 3;", "Error IO"=w1453, "Origin.IOApplication"=w1454) -> ("Error IO Out"=w1451:errorcluster, "Origin.IOApplication"=w1452:refnum<k7>)  [unwired: 1 in, 1 out]
            n902 = local read "Independant Variable:"() -> (w1439:string)
            n903 = stacked-sequence {
              tunnel: w1443 -> [w1469 w1499 w1511 w1533 w1553 w1574 w1595 w1618]
              tunnel: w1442 -> [w1470 w1498 w1512 w1532 w1554 w1575 w1596 w1619]
              tunnel: w1452 -> [w1472 w1496 w1514 w1535 w1556 w1577 w1598 w1621]
              tunnel: w1451 -> [w1471 w1497 w1513 w1534 w1555 w1576 w1597 w1620]
              tunnel: [_ _ _ _ _ _ _ w1616] -> w1441
              tunnel: [_ _ _ _ _ _ _ w1617] -> w1440
              tunnel: w1439 -> [w1468 w1489 w1510 w1531 w1552 w1573 w1594 w1615]
              frame #0 {
                n904 = local read "X Axis Display Type"() -> (w1460:string)
                n905 = local read "Opj X Axis"() -> (w1465:string)
                n906 = Concatenate Strings("window -a MOBLGraph;\nlayer.x.type=", w1465, "; layer.x.label.numFormat = ", w1460, "; Y3 = 1; X3 = 1;", "window -a MOBLTable;\nwindow -s TV;") -> (w1463:string)
                n907 = call "Param_Analysis_7_24b_JW.vi"("Independant Variable"=w1468, "error in (no error)"=w1471, "Data Folder"=w1469, "Parameter String"="Mobility-Lin (cm^2/Vs):", "Parameter Name"="Mobility-Lin", "Stats Folder"=w1470) -> ("error out"=w1474:errorcluster, "Output Array"=w1476:string[][], "Variables"=w1467:T27)  [unwired: 2 in, 1 out]
                n908 = call "Origin_Export_7_27a_JW.vi"("Input Conditions"=w1467, "Analysis Array"=w1476, "error in (no error)"=w1474, "Parameter Worksheet Name"="[MOBLTable]Mobilities", "Parameter Folder Script"="pe_cd \"Mobility-Lin\";", "Origin.IOApplication"=w1472) -> ("error out"=w1473:errorcluster, "reference out"=w1475:refnum<k7>)  [unwired: 3 in, 1 out]
                n909 = call "OAExecute.vi"("script"=w1463, "Error IO"=w1473, "Origin.IOApplication"=w1475) -> ()  [unwired: 1 in, 3 out]
              }
              frame #1 {
                n910 = local read "X Axis Display Type"() -> (w1481:string)
                n911 = local read "Opj X Axis"() -> (w1486:string)
                n912 = Concatenate Strings("window -a MOBSGraph;\nlayer.x.type=", w1486, "; layer.x.label.numFormat = ", w1481, "; Y3 = 1; X3 = 1;", "window -a MOBSTable;\nwindow -s TV;") -> (w1484:string)
                n913 = call "Param_Analysis_7_24b_JW.vi"("Independant Variable"=w1489, "error in (no error)"=w1497, "Data Folder"=w1499, "Parameter String"="Mobility-Sat (cm^2/Vs):", "Parameter Name"="Mobility-Sat", "Stats Folder"=w1498) -> ("error out"=w1492:errorcluster, "Output Array"=w1490:string[][], "Variables"=w1488:T27)  [unwired: 2 in, 1 out]
                n914 = call "Origin_Export_7_27a_JW.vi"("Input Conditions"=w1488, "Analysis Array"=w1490, "error in (no error)"=w1492, "Parameter Worksheet Name"="[MOBSTable]Mobilities", "Parameter Folder Script"="pe_cd \"Mobility-Sat\";", "Origin.IOApplication"=w1496) -> ("error out"=w1491:errorcluster, "reference out"=w1493:refnum<k7>)  [unwired: 3 in, 1 out]
                n915 = call "OAExecute.vi"("script"=w1484, "Error IO"=w1491, "Origin.IOApplication"=w1493) -> ()  [unwired: 1 in, 3 out]
              }
              frame #2 {
                n916 = local read "X Axis Display Type"() -> (w1502:string)
                n917 = local read "Opj X Axis"() -> (w1507:string)
                n918 = Concatenate Strings("window -a NSTSGraph;\nlayer.x.type=", w1507, "; layer.x.label.numFormat = ", w1502, "; Y3 = 1; X3 = 1;", "window -a NSTSTable;\nwindow -s TV;") -> (w1505:string)
                n919 = call "Param_Analysis_7_24b_JW.vi"("Independant Variable"=w1510, "error in (no error)"=w1513, "Data Folder"=w1511, "Parameter String"="Trap Density-STS (Traps/Vcm^2):", "Parameter Name"="Trap Density-STS", "Stats Folder"=w1512) -> ("error out"=w1517:errorcluster, "Output Array"=w1515:string[][], "Variables"=w1509:T27)  [unwired: 2 in, 1 out]
                n920 = call "Origin_Export_7_27a_JW.vi"("Input Conditions"=w1509, "Analysis Array"=w1515, "error in (no error)"=w1517, "Parameter Worksheet Name"="[NSTSTable]Trap Densities", "Parameter Folder Script"="pe_cd \"N-STS\";", "Origin.IOApplication"=w1514) -> ("error out"=w1516:errorcluster, "reference out"=w1518:refnum<k7>)  [unwired: 3 in, 1 out]
                n921 = call "OAExecute.vi"("script"=w1505, "Error IO"=w1516, "Origin.IOApplication"=w1518) -> ()  [unwired: 1 in, 3 out]
              }
              frame #3 {
                n922 = local read "X Axis Display Type"() -> (w1523:string)
                n923 = local read "Opj X Axis"() -> (w1528:string)
                n924 = call "Param_Analysis_7_24b_JW.vi"("Independant Variable"=w1531, "error in (no error)"=w1534, "Data Folder"=w1533, "Parameter String"="Trap Density-VT (Traps/Vcm^2):", "Parameter Name"="Trap Density-Vt", "Stats Folder"=w1532) -> ("error out"=w1538:errorcluster, "Output Array"=w1536:string[][], "Variables"=w1530:T27)  [unwired: 2 in, 1 out]
                n925 = Concatenate Strings("window -a NVtGraph;\nlayer.x.type=", w1528, "; layer.x.label.numFormat = ", w1523, "; Y3 = 1; X3 = 1;", "window -a NVtTable;\nwindow -s TV;") -> (w1526:string)
                n926 = call "Origin_Export_7_27a_JW.vi"("Input Conditions"=w1530, "Analysis Array"=w1536, "error in (no error)"=w1538, "Parameter Worksheet Name"="[NVTTable]Trap Densities", "Parameter Folder Script"="pe_cd \"N-Vt\";", "Origin.IOApplication"=w1535) -> ("error out"=w1537:errorcluster, "reference out"=w1539:refnum<k7>)  [unwired: 3 in, 1 out]
                n927 = call "OAExecute.vi"("script"=w1526, "Error IO"=w1537, "Origin.IOApplication"=w1539) -> ()  [unwired: 1 in, 3 out]
              }
              frame #4 {
                n928 = local read "X Axis Display Type"() -> (w1544:string)
                n929 = local read "Opj X Axis"() -> (w1549:string)
                n930 = Concatenate Strings("window -a OffIGraph;\nlayer.x.type=", w1549, "; layer.x.label.numFormat = ", w1544, "; Y3 = 1; X3 = 1;", "window -a OffITable;\nwindow -s TV;") -> (w1547:string)
                n931 = call "Param_Analysis_7_24b_JW.vi"("Independant Variable"=w1552, "error in (no error)"=w1555, "Data Folder"=w1553, "Parameter String"="Off I-Sat (A):", "Parameter Name"="Off I-Sat", "Stats Folder"=w1554) -> ("error out"=w1559:errorcluster, "Output Array"=w1557:string[][], "Variables"=w1551:T27)  [unwired: 2 in, 1 out]
                n932 = call "Origin_Export_7_27a_JW.vi"("Input Conditions"=w1551, "Analysis Array"=w1557, "error in (no error)"=w1559, "Parameter Worksheet Name"="[OffItable]OffCurrents", "Parameter Folder Script"="pe_cd \"OffI-Sat\";", "Origin.IOApplication"=w1556) -> ("error out"=w1558:errorcluster, "reference out"=w1560:refnum<k7>)  [unwired: 3 in, 1 out]
                n933 = call "OAExecute.vi"("script"=w1547, "Error IO"=w1558, "Origin.IOApplication"=w1560) -> ()  [unwired: 1 in, 3 out]
              }
              frame #5 {
                n934 = local read "X Axis Display Type"() -> (w1565:string)
                n935 = local read "Opj X Axis"() -> (w1570:string)
                n936 = Concatenate Strings("window -a OnOffGraph;\nlayer.x.type=", w1570, "; layer.x.label.numFormat = ", w1565, "; Y3 = 1; X3 = 1;", "window -a OnOffTable;\nwindow -s TV;") -> (w1568:string)
                n937 = call "Param_Analysis_7_24b_JW.vi"("Independant Variable"=w1573, "error in (no error)"=w1576, "Data Folder"=w1574, "Parameter String"="On/Off I-Sat:", "Parameter Name"="OnOff Ratio", "Stats Folder"=w1575) -> ("error out"=w1580:errorcluster, "Output Array"=w1578:string[][], "Variables"=w1572:T27)  [unwired: 2 in, 1 out]
                n938 = call "Origin_Export_7_27a_JW.vi"("Input Conditions"=w1572, "Analysis Array"=w1578, "error in (no error)"=w1580, "Parameter Worksheet Name"="[OnOffTable]On/Off Ratios", "Parameter Folder Script"="pe_cd \"OnOff-Ratio\";", "Origin.IOApplication"=w1577) -> ("error out"=w1579:errorcluster, "reference out"=w1581:refnum<k7>)  [unwired: 3 in, 1 out]
                n939 = call "OAExecute.vi"("script"=w1568, "Error IO"=w1579, "Origin.IOApplication"=w1581) -> ()  [unwired: 1 in, 3 out]
              }
              frame #6 {
                n940 = local read "X Axis Display Type"() -> (w1586:string)
                n941 = local read "Opj X Axis"() -> (w1591:string)
                n942 = call "Param_Analysis_7_24b_JW.vi"("Independant Variable"=w1594, "error in (no error)"=w1597, "Data Folder"=w1595, "Parameter String"="STS-Sat (V/decade):", "Parameter Name"="STS-Sat", "Stats Folder"=w1596) -> ("error out"=w1601:errorcluster, "Output Array"=w1599:string[][], "Variables"=w1593:T27)  [unwired: 2 in, 1 out]
                n943 = Concatenate Strings("window -a SGraph;\nlayer.x.type=", w1591, "; layer.x.label.numFormat = ", w1586, "; Y3 = 1; X3 = 1;", "window -a STable;\nwindow -s TV;") -> (w1589:string)
                n944 = call "Origin_Export_7_27a_JW.vi"("Input Conditions"=w1593, "Analysis Array"=w1599, "error in (no error)"=w1601, "Parameter Worksheet Name"="[STable]Threshold Swing", "Parameter Folder Script"="pe_cd \"STS-Sat\";", "Origin.IOApplication"=w1598) -> ("error out"=w1600:errorcluster, "reference out"=w1602:refnum<k7>)  [unwired: 3 in, 1 out]
                n945 = call "OAExecute.vi"("script"=w1589, "Error IO"=w1600, "Origin.IOApplication"=w1602) -> ()  [unwired: 1 in, 3 out]
              }
              frame #7 {
                n946 = local read "X Axis Display Type"() -> (w1607:string)
                n947 = local read "Opj X Axis"() -> (w1612:string)
                n948 = Concatenate Strings("window -a VtGraph;\nlayer.x.type=", w1612, "; layer.x.label.numFormat = ", w1607, "; Y3 = 1; X3 = 1;", "window -a VtTable;\nwindow -s TV;") -> (w1610:string)
                n949 = call "Param_Analysis_7_24b_JW.vi"("Independant Variable"=w1615, "error in (no error)"=w1620, "Data Folder"=w1618, "Parameter String"="Vt-Sat (V):", "Parameter Name"="Vt-Sat", "Stats Folder"=w1619) -> ("error out"=w1624:errorcluster, "Output Array"=w1622:string[][], "Variables"=w1614:T27)  [unwired: 2 in, 1 out]
                n950 = call "Origin_Export_7_27a_JW.vi"("Input Conditions"=w1614, "Analysis Array"=w1622, "error in (no error)"=w1624, "Parameter Worksheet Name"="[VtTable]Threshold Voltages", "Parameter Folder Script"="pe_cd \"Vt-Sat\";", "Origin.IOApplication"=w1621) -> ("error out"=w1623:errorcluster, "reference out"=w1625:refnum<k7>)  [unwired: 3 in, 1 out]
                n951 = call "OAExecute.vi"("script"=w1610, "Error IO"=w1623, "Origin.IOApplication"=w1625) -> ("Error IO Out"=w1616:errorcluster, "Origin.IOApplication"=w1617:refnum<k7>)  [unwired: 1 in, 1 out]
              }
            }
            n952 = Path To String(path=w1446) -> (string=w1445:string)
            n953 = call "OAExecute.vi"("script"="pe_cd /; ", "Error IO"=w1441, "Origin.IOApplication"=w1440) -> ("Error IO Out"=w1447:errorcluster, "Origin.IOApplication"=w1448:refnum<k7>)  [unwired: 1 in, 1 out]
            n954 = call <userlib>:"OASaveProject.vi"("path"=w1445, "Error IO"=w1447, "Origin.IOApplication"=w1448) -> ()  [unwired: 3 out]
          }
        }
      }
    }
    "Current State" <- w15
    "Folder Index" <- w27
    n955 = Wait (ms)(milliseconds to wait=w21) -> ()  [unwired: 1 out]
    n956 = Equal?(x=w12, y=MegaAwesome_States."Exit") -> (x = y?=w14:bool)
  }
  n957 = call "Close LabView?"("Enable"=w2) -> ("OK"=w1:bool)  [unwired: 17 in, 1 out]
  n958 = Quit LabVIEW(quit? (T)=w1) -> ()
